vi "WHD_VEten_0.1.3.WS_BIDIR_Calibr_2.vi"() -> ()   [LabVIEW 2015]
uses:
  <vilib>/NI_Real-Time Target Support.lvlib
  <vilib>/rvi/interface/nirviReadWriteControl/nirviReadWriteControl.xnode
  <vilib>/rvi/interface/nirviMethod/nirviMethod.xnode
  <vilib>/rvi/interface/nirviOpenFPGA/nirviOpenFPGA.xnode
  <vilib>/rvi/interface/nirviCloseFPGA/nirviCloseFPGA.xnode
  <vilib>/userdefined/High Color/nirio_resource_hc.ctl
  <vilib>/rvi/errors/niLvFpgaMergeErrorWithErrorCode.vi
  <vilib>/Utility/file.llb/Write Delimited Spreadsheet (string).vi
  <vilib>/RTwatchdog.llb/Watchdog expiration actions.ctl
  AURA_Wheel/Json2Labv.lvlib
  AURA_Wheel/AuraWheelAPI/AuraWheel.lvlib
  <vilib>/rvi/errors/niLvFpgaAdjustHostInterfaceError.vi
  NiFpgaLv.dll
  <vilib>/Utility/error.llb/Error Cluster From Error Code.vi
  <vilib>/LabVIEW Targets/FPGA/cRIO/shared/nicrio_ModuleControls/nicrio_cRIO-9234_DataRatesRing2.ctl
  <vilib>/FPGAPlugInAG/cRIO-9031/niLvFpga_Run_cRIO-9031.vi
  <vilib>/FPGAPlugInAG/cRIO-9031/niLvFpga_Reset_cRIO-9031.vi
  FPGA Bitfiles/W&RDArabia_FPGATarget_FPGA8a2wsBIdirec_yJvL9yuTbZw.lvbitx
  <vilib>/Utility/config.llb/NI_LVConfig.lvlib
  <vilib>/Utility/config.llb/Write Key (Double).vi
  <vilib>/FPGAPlugInAG/cRIO-9031/niLvFpga_Open_cRIO-9031.vi
  <vilib>/FPGAPlugInAG/cRIO-9031/niLvFpga_ConfigureFifo_cRIO-9031.vi
  <vilib>/FPGAPlugInAG/cRIO-9031/niLvFpga_StartFifo_cRIO-9031.vi
  <vilib>/FPGAPlugInAG/cRIO-9031/niLvFpga_ReadFifo_cRIO-9031.vi
  <vilib>/FPGAPlugInAG/cRIO-9031/niLvFpga_StopFifo_cRIO-9031.vi
  <vilib>/FPGAPlugInAG/cRIO-9031/niLvFpga_Close_cRIO-9031.vi
panel:
  in  "Developer commad":string
  out "Save calibration":bool
  out "calibration log":path
  out "Pattern amplitude (g)":dbl=1.02
  out "Pattern frequency (Hz)":dbl=159.2
  out "Folder":path
  out "Report":string
  out "path calib":path
  out "AURA wheel test":bool
  out "LOG.txt":path
  out "Report_AURA":string
  out "RFID_Error":errorcluster
  out "error FPGA":errorcluster
  out "error AURA":errorcluster
  out "error manipulacion archivos":errorcluster
  out "Response headers":string
  out "Max RMS Ruedas":dbl[][](array[numeric])
  out "TAGs LR6":string[](array[string])
  out "TAGs HEX":string[](array[string])
  out "Parar":bool
  out "result":bool
  out "TAGs":string[](array[string])
  out "Temperatura (ºC)":dbl
  out "V (m/s)":dbl
  out "Digital?":bool=TRUE
  out "Watchdog config":T1={"reset system"=FALSE, "restart LabVIEW Runtime"=FALSE, "occurrence"=FALSE, "trigger protocol"=enum."active high", "trigger line"=enum."none", "disable watchdog on VI exit"=TRUE}
  out "Tiempo de adquisicion":dbl=10.0
  out "Adquirir":bool
  out "Nº Ruedas 1":i32
  out "NºRuedas 2":i32
  out "Disco Duro Disponible (bytes)":i64
  out "Buffer Overflow":bool
  out "Buffer Underflow":bool
  out "Archivo\nvalido?":bool
  out "Número de ejes detectados":i32
  out "Ejes_convoy":i32
  out "Tiempo de paso (s)":dbl
  out "created path":path
  out "Nombre de archivo":path[](array[path])
  out "LR6 IP address":string="192.168.106.94"
  out "Port LR6":u16=2001
  out "T fuera rango":bool
  out "Frecuencia de muestreo (Hz)":dbl=25600.0
  out "Escaneos de la FIFO por canal":u32=5000
  out "Tiempo extra al detector de paso (s)":dbl=1.0
  out "dt RMS":dbl=256.0
  out "Frecuencia de muestreo y módulo CRIO":T2=2 items=["51.200 kS/s (NI 9234)"=1, "25.600 kS/s (NI 9234)"=2, "17.067 kS/s (NI 9234)"=3, "12.800 kS/s (NI 9234)"=4, "10.240 kS/s (NI 9234)"=5, "8.533 kS/s (NI 9234)"=6, "7.314 kS/s (NI 9234)"=7, "6.400 kS/s (NI 9234)"=8, "5.689 kS/s (NI 9234)"=9, "5.120 kS/s (NI 9234)"=10, "4.654 kS/s (NI 9234)"=11, "4.267 kS/s (NI 9234)"=12, "3.938 kS/s (NI 9234)"=13, "3.657 kS/s (NI 9234)"=14, "3.413 kS/s (NI 9234)"=15, "3.200 kS/s (NI 9234)"=16, "3.012 kS/s (NI 9234)"=17, "2.845 kS/s (NI 9234)"=18, "2.695 kS/s (NI 9234)"=19, "2.560 kS/s (NI 9234)"=20, "2.438 kS/s (NI 9234)"=21, "2.328 kS/s (NI 9234)"=22, "2.226 kS/s (NI 9234)"=23, "2.133 kS/s (NI 9234)"=24, "2.048 kS/s (NI 9234)"=25, "1.969 kS/s (NI 9234)"=26, "1.896 kS/s (NI 9234)"=27, "1.829 kS/s (NI 9234)"=28, "1.765 kS/s (NI 9234)"=29, "1.707 kS/s (NI 9234)"=30, "1.652 kS/s (NI 9234)"=31]
  out "Puerto RFID":u16=2189
  out "IP RFID":string="192.168.106.99"
  out "Offset_rueda WS 2":fxp<+/-,24,-4>=0.004999998956918716 format="%.27g"
  out "Count(mSec)":u32=2
  out "RFID NEM on?":bool
  out "RFID LR6 on?":bool
  out "Canal cero WS1?":bool
  out "Canal cero WS2":bool
  out "Inicio pasada 2":timestamp
  in  "Calibration":bool
  out "Direccion 0?":bool
  out "Boton Adquirir?":bool
  out "RuedaDetectada2?":bool=TRUE
  out "RuedaDetectada1?":bool=TRUE
  out "Timeout ruedas":dbl
  out "Borrar archivos\nadquisicion con error":bool
  out "Able watchdog?":bool
  out "Reset watchdog?":bool
  out "Leer config RFID NEM":bool
  out "bytes to read":i32
  out "DeviceAddress":u8
  out "timeout ms (60000)":i32
  out "Max archivos":u32=2
  out "Bytes libre despues de borrar":u32=2
  out "Bytes min libre":u32=2
  out "Nº de acelerómetros":i32
  out "Nº inductivos":i32
  out "Offset_rueda WS 1":fxp<+/-,24,-4>=0.004999998956918716 format="%.27g"
  out "TAGs_AURAwheel":string[][](array[string])
  out "Plataformas?":bool
  out "Nº Ejes":i32[](array[numeric])
  out "Nº UTs":i32
  out "it-read-LR6":i32[](array[numeric])
  out "it-LR6":i32
  out "RFID_LR6_Error":errorcluster
  out "Series_flota":string[](array[string])
  out "Tabla_flota":string[][](array[string])
  out "Puntos medios de las ventanas":dbl[][](array[numeric])
  out "configuration file path":path=path "c:/Parametros.cfg"
  out "IP synchr":string
  out "data":cluster{"status":string}
  out "confRFID":path=path "c:/RFID/TAGS.csv"
  out "TAGS leidos":path=path "c:/RFID/TAGS.csv"
  out "Use Aura?":bool
  out "Parametros AuraWheel":string[](array[string])
  out "Parámetros acelerómetros":dbl[](array[numeric])
  out "Fin":bool
  out "Contador":i32=1
  out "Path LOG":path=path "c:/TEST"
  out "Fallo fotocelula":bool
  out "Path_Borrar":path=path "c:/Trenes"
  out "Longitud de la unidad":dbl
  out "Aviso no detección":string
  out "Time to Acquire Block (ms)":i32
  out "Distancia de acelerómetros":dbl[](array[numeric])
  out "Block Size":u32
  out "Distancias generales":dbl[](array[numeric])
  out "Reset del controlador":bool
  out "Parar la aplicación":bool
  out "date/time string":string
  out "Timeout ruedas":bool
  out "Tiempo":dbl
  out "Inicio pasada":timestamp
  out "Ultimo TEST":timestamp
  out "Fuente":bool=TRUE
  out "RFID_ID":refnum<k5>
  out "DC OK":string
  out "Aviso temperatura":string
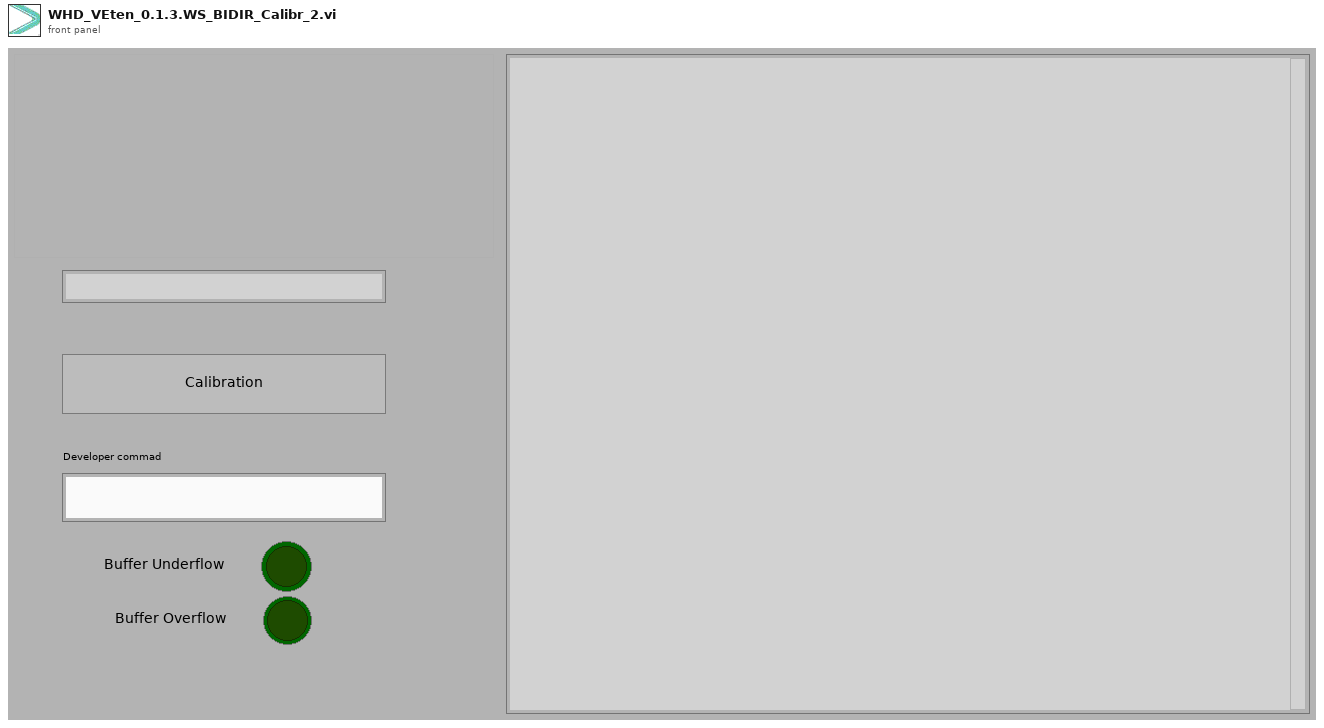
[diagram p1: front panel]
types:
  T1 = typedef "Watchdog expiration actions.ctl" = cluster{"reset system":bool, "restart LabVIEW Runtime":bool, "occurrence":bool, "trigger protocol":enum16{"active high", "active low", "open collector"}, "trigger line":enum16{"none", "line 0", "line 1", "line 2", "line 3", "line 4", "line 5", "line 6", "line 7", "SMB line 0"}, "disable watchdog on VI exit":bool}
  T2 = typedef "nicrio_cRIO-9234_DataRatesRing2.ctl" = u8
  T3 = typedef "nirio_resource_hc.ctl" = tag
  T4 = enum16{"Standard", "Buffered", "CRLF", "Immediate"}
  T5 = enum16{"open", "replace", "create", "open or create", "replace or create", "replace or create with confirmation"}
  T6 = enum16{"big-endian, network order", "native, host order", "little-endian"}
  T7 = cluster{"error IO":errorcluster, bool[], u32[], string[], dbl[]}
  T8 = cluster{"error out":errorcluster, dbl[], "TAGs":string[], "Direccion 0?":bool}
  T9 = cluster{"g_ts":dbl, "p_sp":dbl, "p_tp":dbl, "p_tg":cluster{"tg_n":dbl, "tg_t":string}[], "p_ax":cluster{"ax_n":dbl, "ax_sp":dbl, "ax_wh":cluster{"wh_p":dbl, "wh_a1":dbl, "wh_a2":dbl, "wh_a3":dbl, "wh_a4":dbl}[]}[]}
  T10 = cluster{"Frecuencia de muestreo y módulo CRIO":T2, "Count(mSec)":u32, "Frecuencia de muestreo (Hz)":dbl, "Escaneos de la FIFO por canal":u32, "Nº inductivos":i32, "Nº de acelerómetros":i32}
  T11 = typedef "NI_LVConfig.lvlib/Config Data RefNum.ctl" = refnum<k1>
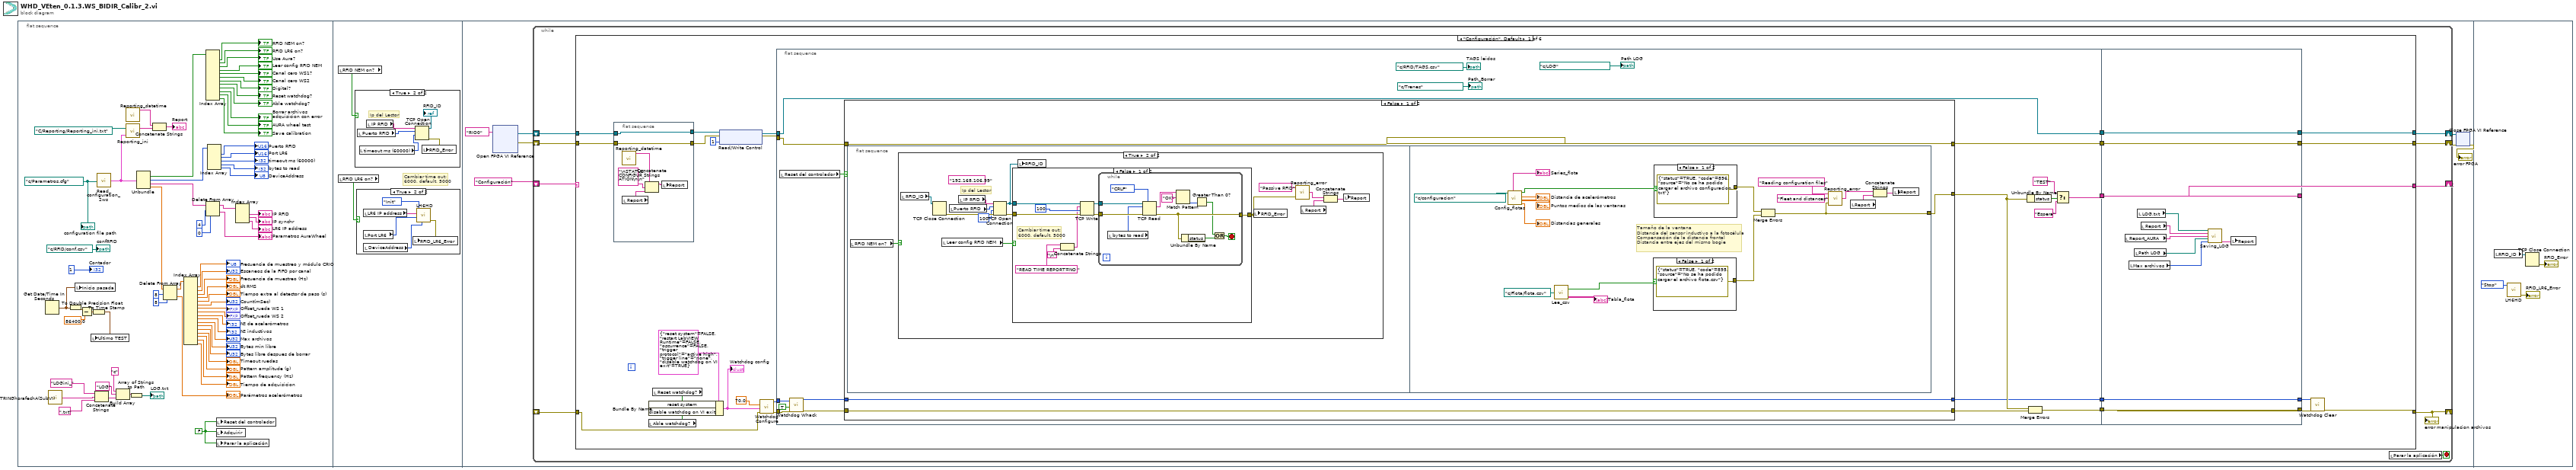
[diagram p0: block diagram]
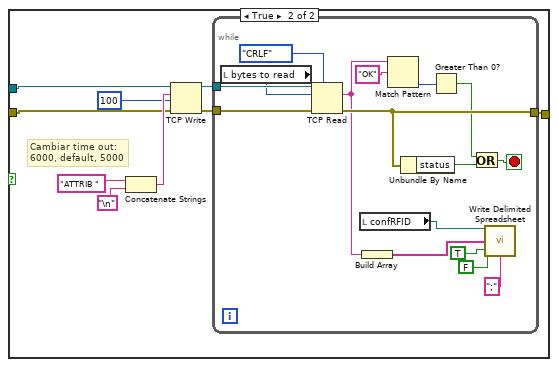
[diagram p5: hidden frame]
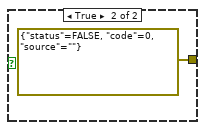
[diagram p6: hidden frame]
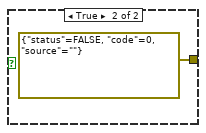
[diagram p7: hidden frame]
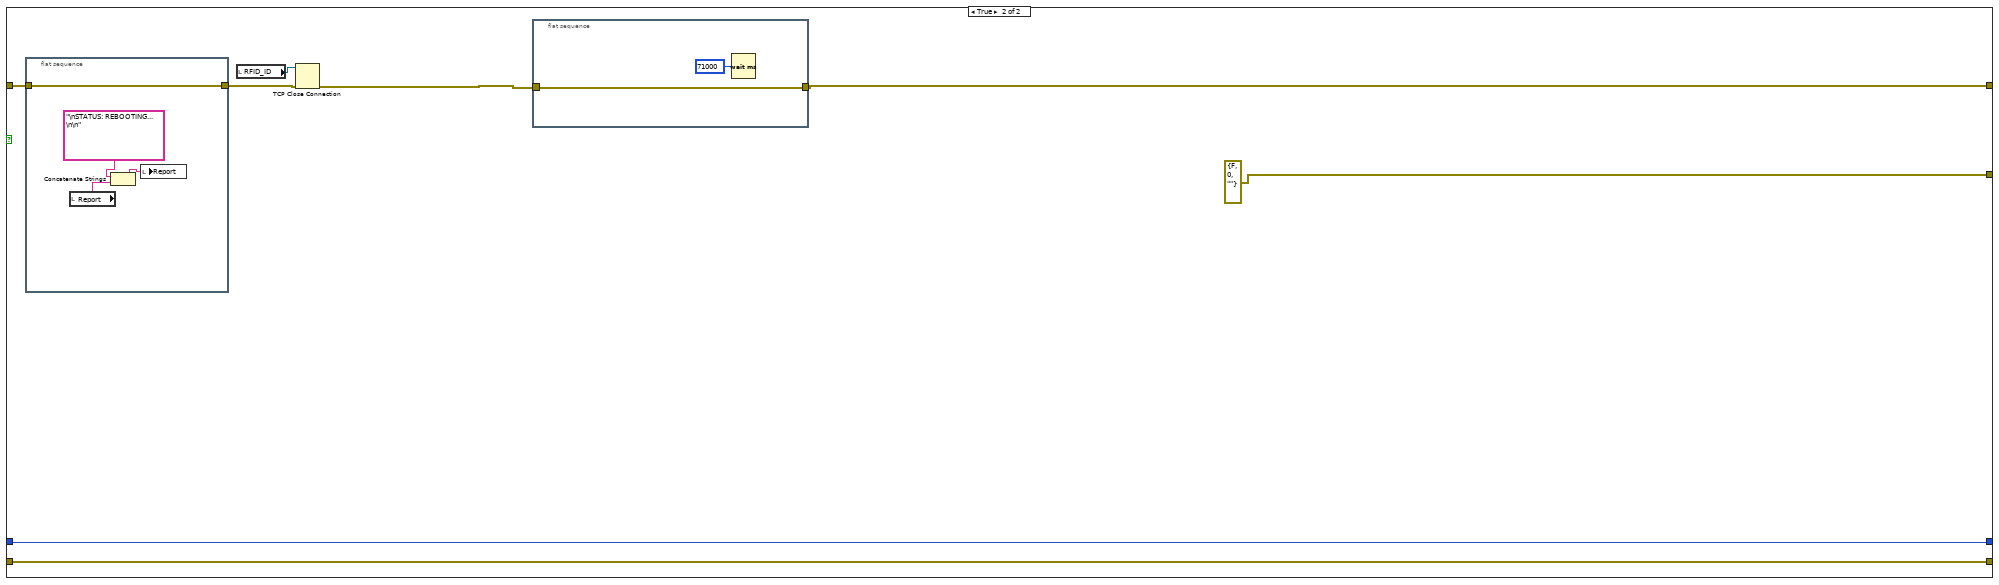
[diagram p8: hidden frame]
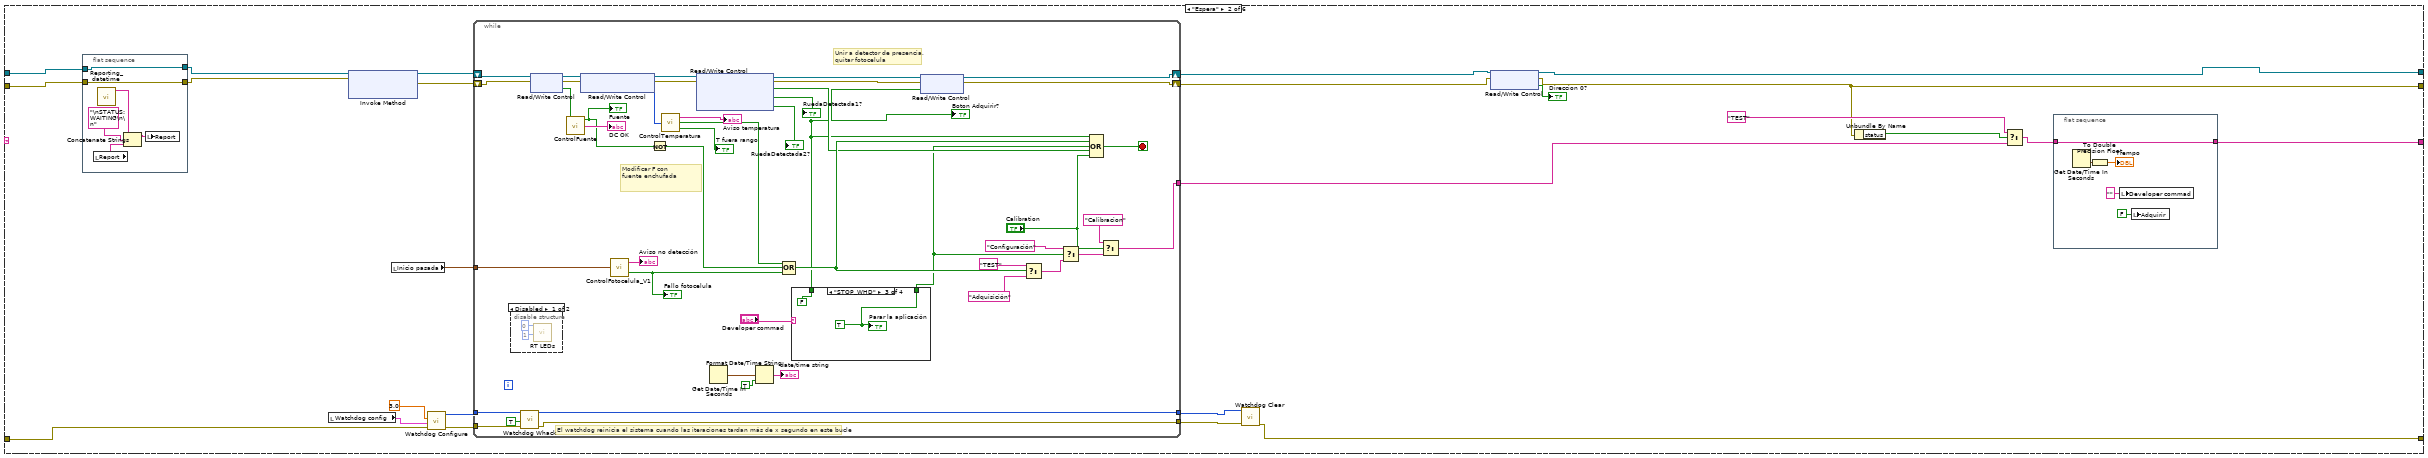
[diagram p9: hidden frame]
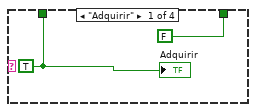
[diagram p10: hidden frame]
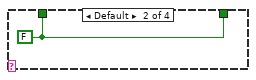
[diagram p11: hidden frame]
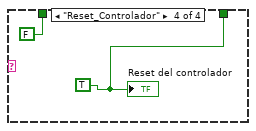
[diagram p12: hidden frame]
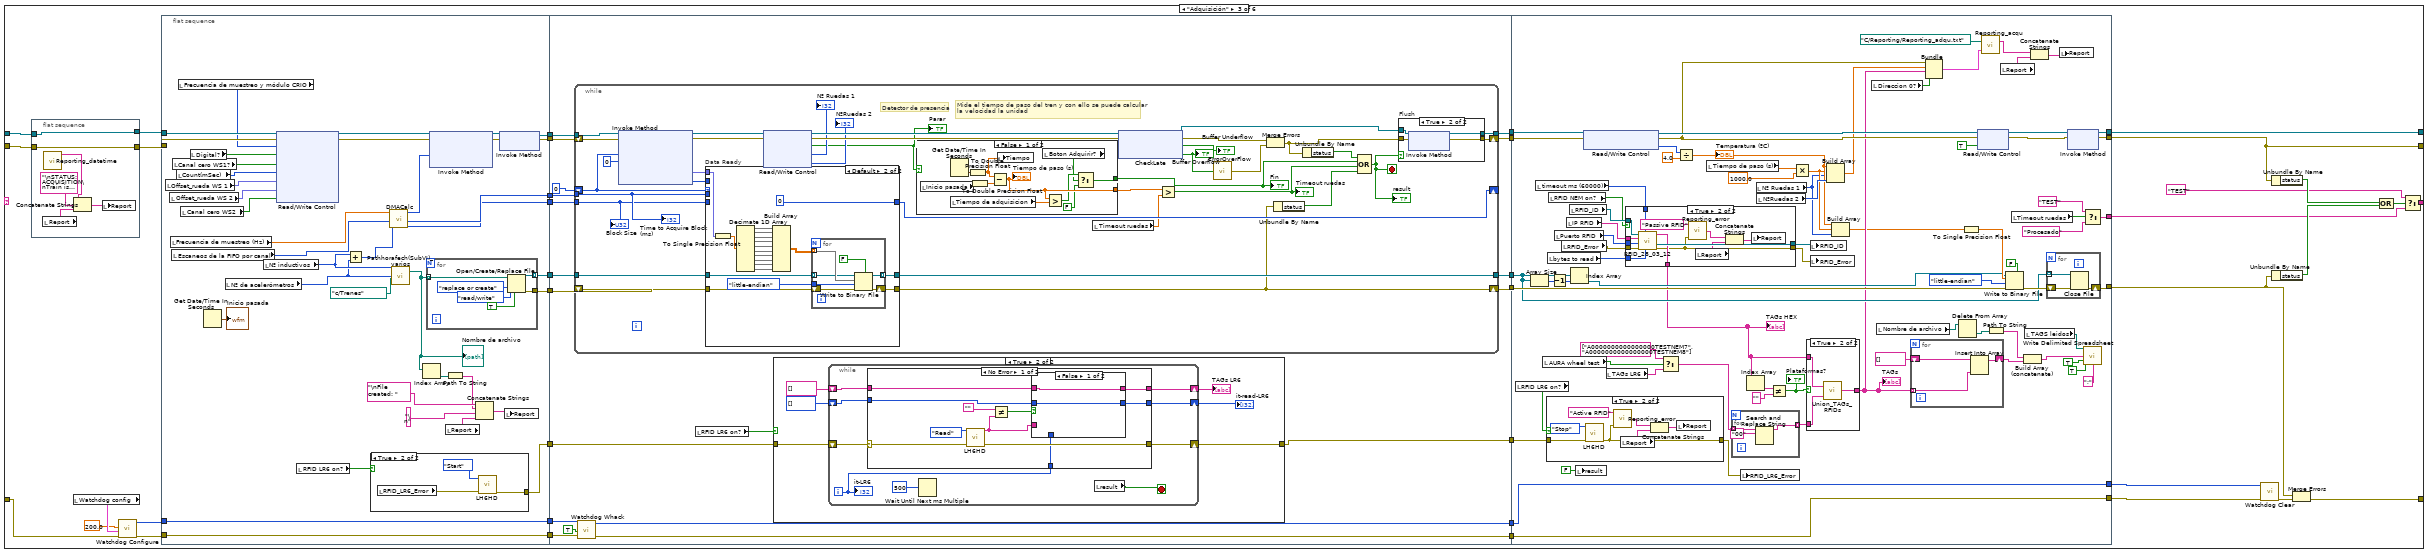
[diagram p14: hidden frame]
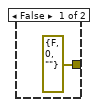
[diagram p15: hidden frame]
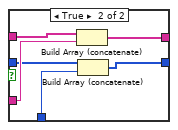
[diagram p17: hidden frame]
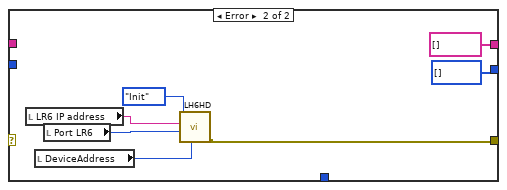
[diagram p18: hidden frame]
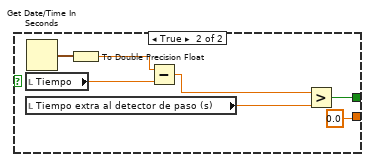
[diagram p19: hidden frame]
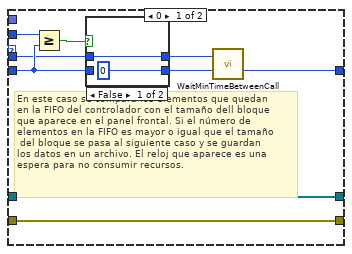
[diagram p20: hidden frame]
diagram:
  n1 = flat-sequence {
    frame #0 {
      w1 = FALSE ("Reset del controlador")
      w63 = path "c:/Parametros.cfg" ("configuration file path")
      n2 = Get Date/Time In Seconds() -> (seconds since 1Jan1904=w68:timestamp)
      n3 = call "STRINGhorafechA(SubVI).vi"() -> ("STRINGhora_fecha"=w12:string)
      n4 = To Double Precision Float(number=w68) -> (double precision float=w70:dbl)
      n5 = local write "Inicio pasada"(w68) -> ()
      n6 = Subtract(x=w70, y=86400.0) -> (x-y=w69:dbl)
      n7 = To Time Stamp(1:w69) -> (0:w67:timestamp)
      n8 = local write "Ultimo TEST"(w67) -> ()
      n9 = Concatenate Strings("LOGini_" ("string"), w12, ".txt" ("string")) -> (w14:string)
      n10 = call "Read_configuration_2ws.vi"("configuration file path"=w63) -> ("output cluster"=w18:T7)
      n11 = Build Array("c", "LOG" ("element"), w14) -> (w11:string[])
      n12 = call "Reporting_ini.vi"("Configuration cluster"=w18, "address repoting"=path "C:/Reporting/Reporting_ini.txt" ("file (use dialog)")) -> ("Reporting"=w17:string)  [unwired: 1 in]
      n13 = call "Reporting_datetime.vi"() -> ("String"=w15:string)  [unwired: 11 in]
      n14 = Array of Strings to Path(0:w11) -> (2:→"LOG.txt":path)  [unwired: 1 out]
      n15 = Unbundle(w18) -> (w66:bool[], w65:u32[], w58:string[], w62:dbl[])  [unwired: 1 out]
      n16 = Concatenate Strings(w15, w17) -> (→"Report":string)
      n17 = Delete From Array(array=w62, length=8, index=8) -> (deleted portion=→"Parámetros acelerómetros":dbl[], array with subset deleted=w61:dbl[])
      n18 = Index Array(array=w61) -> (element #1=→"Frecuencia de muestreo y módulo CRIO":dbl, element #2=→"Escaneos de la FIFO por canal":dbl, element #3=→"Frecuencia de muestreo (Hz)":dbl, element #4=→"dt RMS":dbl, element #5=→"Tiempo extra al detector de paso (s)":dbl, element #6=→"Count(mSec)":dbl, element #7=→"Offset_rueda WS 1":dbl, element #8=→"Offset_rueda WS 2":dbl, element #9=→"Nº de acelerómetros":dbl, element #10=→"Nº inductivos":dbl, element #11=→"Max archivos":dbl, element #12=→"Bytes min libre":dbl, element #13=→"Bytes libre despues de borrar":dbl, element #14=→"Timeout ruedas":dbl, element #15=→"Pattern amplitude (g)":dbl, element #16=→"Pattern frequency (Hz)":dbl, element #17=→"Tiempo de adquisicion":dbl)  [unwired: 17 in]
      n19 = Index Array(array=w66) -> (element #1=→"RFID NEM on?":bool, element #2=→"RFID LR6 on?":bool, element #3=→"Use Aura?":bool, element #4=→"Leer config RFID NEM":bool, element #5=→"Canal cero WS1?":bool, element #6=→"Canal cero WS2":bool, element #7=→"Digital?":bool, element #8=→"Reset watchdog?":bool, element #9=→"Able watchdog?":bool, element #10=→"Borrar archivos\nadquisicion con error":bool, element #11=→"AURA wheel test":bool, element #12=→"Save calibration":bool)  [unwired: 12 in]
      n20 = Delete From Array(array=w58, length=4, index=0) -> (deleted portion=→"Parametros AuraWheel":string[], array with subset deleted=w57:string[])
      n21 = Index Array(array=w65) -> (element #1=→"Puerto RFID":u32, element #2=→"Port LR6":u32, element #3=→"timeout ms (60000)":u32, element #4=→"bytes to read":u32, element #5=→"DeviceAddress":u32)  [unwired: 5 in]
      n22 = local write "Reset del controlador"(w1) -> ()
      n23 = local write "Adquirir"(w1) -> ()
      n24 = local write "Parar la aplicación"(w1) -> ()
      n25 = Index Array(array=w57) -> (element #1=→"IP RFID":string, element #2=→"IP synchr":string, element #3=→"LR6 IP address":string)  [unwired: 3 in]
      "Contador" <- 1
      "confRFID" <- path "c:/RFID/conf.csv" ("file path (use dialog)")
      "configuration file path" <- w63
    }
    frame #1 {
      # "Cambiar time out:\n6000, default, 5000"
      n26 = local read "RFID NEM on?"() -> (w73:bool)
      n27 = local read "RFID LR6 on?"() -> (w72:bool)
      n28 = case shown="True" w73 {
        frame False {
        }
        frame True {
          # "Ip del Lector"
          n29 = local read "Puerto RFID"() -> (w81:u16)
          n30 = local read "timeout ms (60000)"() -> (w79:i32)
          n31 = local read "IP RFID"() -> (w82:string)
          n32 = TCP Open Connection(address=w82, remote port or service name=w81, timeout ms (60000)=w79) -> (connection ID=→"RFID_ID":refnum<k5>, error out=w80:errorcluster)  [unwired: 1 in, 1 out]
          n33 = local write "RFID_Error"(w80) -> ()
        }
      }
      n34 = case shown="True" w72 {
        frame False {
        }
        frame True {
          n35 = local read "LR6 IP address"() -> (w74:string)
          n36 = local read "Port LR6"() -> (w75:u16)
          n37 = local read "DeviceAddress"() -> (w76:u8)
          n38 = call "LH6HD.vi"("DeviceAddress"=w76, "Reader Port"=w75, "IP Address"=w74, "Action"=enum16{"Init", "Start", "Read", "Stop", "Exit"}."Init") -> ("error out"=w78:errorcluster)  [unwired: 6 in, 1 out]
          n39 = local write "RFID_LR6_Error"(w78) -> ()
        }
      }
    }
    frame #2 {
      n40 = xnode "Open FPGA VI Reference"("resource name"=T3 "RIO0") -> ("FPGA VI Reference Out"=w90:refnum<k20>, "error out"=w89:errorcluster)  [unwired: 1 in]
      n41 = while {
        shift-right: [w91] -> _
        shift-left: "Configuración" -> [w99]
        shift-right: [w93] -> w86
        shift-left: w90 -> [w98]
        shift-right: [w92] -> w85
        shift-left: w89 -> [w97]
        shift-right: [w96] -> _
        shift-left: _ -> [w95]
        stop <- w94 stop-if-true
        n42 = case shown="\"Configuración\", Default" w99 {
          tunnel: [w114 w278 w368 w725 w973 "Espera"] -> w91
          tunnel: [w124 w266 w382 w714 w972 w1046] -> w93
          tunnel: [w125 w265 w383 w712 w971 w1045] -> w92
          tunnel: w98 -> [w108 w264 w354 w715 w972 w1051]
          tunnel: w97 -> [w107 w263 w353 w713 w964 w1050]
          tunnel: [w121 w272 w380 w710 w963 _] -> w96
          tunnel: w95 -> [w113 w277 w364 w724 w960 _]
          frame "Configuración", Default {
            n43 = flat-sequence {
              tunnel: w108 -> [w131]
              tunnel: w107 -> [w130]
              tunnel: [w131] -> w106
              tunnel: [w130] -> w105
              frame #0 {
                n44 = call "Reporting_datetime.vi"() -> ("String"=w126:string)  [unwired: 11 in]
                n45 = local read "Report"() -> (w127:string)
                n46 = Concatenate Strings(w126, "\nSTATUS: CONFIGURATION\n\n", w127) -> (w129:string)
                n47 = local write "Report"(w129) -> ()
              }
            }
            n48 = local read "Able watchdog?"() -> (w118:bool)
            n49 = local read "Reset watchdog?"() -> (w119:bool)
            n50 = Bundle By Name(cluster=T1 {"reset system"=FALSE, "restart LabVIEW Runtime"=FALSE, "occurrence"=FALSE, "trigger protocol"=enum."active high", "trigger line"=enum."none", "disable watchdog on VI exit"=TRUE} ("expiration actions"), "reset system"=w119, "disable watchdog on VI exit"=w118) -> (w112:T1)
            "Watchdog config" <- w112
            n51 = xnode "Read/Write Control"("FPGA VI Reference In"=w106, "error in"=w105, "Cycles to Filter"=u16 1) -> ("FPGA VI Reference Out"=w117:refnum<k20>, "error out"=w116:errorcluster)
            n52 = call <vilib>:"Watchdog Configure.vi"("error in (no error)"=w113, "expiration actions"=w112, "timeout (1 sec)"=70.0) -> ("error out"=w109:errorcluster, "watchdogID"=w110:u64)  [unwired: 1 in, 2 out]
            n53 = flat-sequence {
              tunnel: w117 -> [w143]
              tunnel: w116 -> [w140]
              tunnel: w110 -> [w133]
              tunnel: w109 -> [w132]
              tunnel: [w142] -> w104
              tunnel: [w150] -> w103
              tunnel: [w143] -> w102
              tunnel: [w145] -> w101
              tunnel: [w137] -> w100
              tunnel: [w256] -> w123
              tunnel: [w257] -> w122
              tunnel: [w258] -> w124
              tunnel: [w259] -> w114
              tunnel: [w260] -> w125
              tunnel: w104 -> [w260]
              tunnel: w103 -> [w259]
              tunnel: w102 -> [w258]
              tunnel: w101 -> [w257]
              tunnel: w100 -> [w256]
              frame #0 {
                n54 = local read "Reset del controlador"() -> (w139:bool)
                n55 = call <vilib>:"Watchdog Whack.vi"("error in (no error)"=w132, "reset watchdog after expire? (F)"=TRUE, "watchdogID in"=w133) -> ("error out"=w135:errorcluster, "watchdogID out"=w136:u64)  [unwired: 2 in, 1 out]
                n56 = case shown="False" w139 {
                  tunnel: w140 -> [w155 w238]
                  tunnel: [w155 w241] -> w142
                  tunnel: [w152 errorcluster {"status"=FALSE, "code"=0, "source"=""} ("error IO")] -> w141
                  tunnel: [w154 w240] -> w137
                  tunnel: w136 -> [w154 w240]
                  tunnel: w135 -> [w153 w239]
                  tunnel: [w153 w239] -> w134
                  frame False {
                    n57 = flat-sequence {
                      tunnel: [w215] -> w152
                      frame #0 {
                        n58 = local read "RFID NEM on?"() -> (w156:bool)
                        n59 = case shown="True" w156 {
                          frame False {
                          }
                          frame True {
                            (unwired) "192.168.106.99" ("address")
                            # "Ip del Lector"
                            n60 = local read "RFID_ID"() -> (w168:refnum<k5>)
                            n61 = TCP Close Connection(connection ID=w168) -> (error out=w169:errorcluster)  [unwired: 2 in, 1 out]
                            n62 = local read "Leer config RFID NEM"() -> (w162:bool)
                            n63 = local read "Puerto RFID"() -> (w166:u16)
                            n64 = local read "IP RFID"() -> (w165:string)
                            n65 = TCP Open Connection(address=w165, remote port or service name=w166, timeout ms (60000)=100, error in (no error)=w169) -> (connection ID=w167:refnum<k5>, error out=w163:errorcluster)  [unwired: 1 out]
                            n66 = case shown="False" w162 {
                              tunnel: w167 -> [w178 w192]
                              tunnel: [w176 w190] -> w161
                              tunnel: w163 -> [w173 w191]
                              frame False {
                                # "Cambiar time out:\n6000, default, 5000"
                                n67 = Concatenate Strings("READ TIME REPORT=NO " ("data in"), "\n") -> (w170:string)
                                n68 = TCP Write(connection ID=w178, data in=w170, error in (no error)=w173, 9:100 ("timeout ms (25000)")) -> (connection ID out=w174:refnum<k5>, error out=w175:errorcluster)  [unwired: 1 out]
                                n69 = while {
                                tunnel: w175 -> [w188]
                                tunnel: w174 -> [w187]
                                tunnel: [w186] -> w176
                                stop <- w183 stop-if-true
                                n70 = local read "bytes to read"() -> (w179:i32)
                                n71 = TCP Read(connection ID=w187, bytes to read=w179, error in (no error)=w188, 7:T4."CRLF" ("mode (standard)")) -> (data out=w181:string, error out=w186:errorcluster)  [unwired: 1 in, 1 out]
                                n72 = Match Pattern(string=w181, regular expression="OK") -> (offset past match=w184:i32)  [unwired: 4 out]
                                n73 = Unbundle By Name(w186) -> ("status"=w182:bool)
                                n74 = Greater Than 0?(x=w184) -> (x > 0?=w180:bool)
                                n75 = Or(x=w180, y=w182) -> (x .or. y?=w183:bool)
                                }
                              }
                              frame True {
                                # "Cambiar time out:\n6000, default, 5000"
                                n76 = Concatenate Strings("ATTRIB " ("data in"), "\n") -> (w198:string)
                                n77 = TCP Write(connection ID=w192, data in=w198, error in (no error)=w191, 9:100 ("timeout ms (25000)")) -> (connection ID out=w195:refnum<k5>, error out=w194:errorcluster)  [unwired: 1 out]
                                n78 = while {
                                tunnel: w194 -> [w213]
                                tunnel: w195 -> [w212]
                                tunnel: [w211] -> w190
                                stop <- w208 stop-if-true
                                n79 = local read "bytes to read"() -> (w199:i32)
                                n80 = TCP Read(connection ID=w212, bytes to read=w199, error in (no error)=w213, 7:T4."CRLF" ("mode (standard)")) -> (data out=w202:string, error out=w211:errorcluster)  [unwired: 1 in, 1 out]
                                n81 = local read "confRFID"() -> (w201:path)
                                n82 = Build Array(w202) -> (w200:string[])
                                n83 = Match Pattern(string=w202, regular expression="OK") -> (offset past match=w209:i32)  [unwired: 4 out]
                                n84 = Unbundle By Name(w211) -> ("status"=w207:bool)
                                n85 = Greater Than 0?(x=w209) -> (x > 0?=w206:bool)
                                n86 = Or(x=w206, y=w207) -> (x .or. y?=w208:bool)
                                n87 = call-poly <vilib>:"Write Delimited Spreadsheet.vi"("file path (dialog if empty)"=w201, "1D data"=w200, "append to file? (new file:F)"=FALSE ("transpose? (no:F)"), "transpose? (no:F)"=TRUE ("append to file? (new file:F)"), "delimiter (\\t)"=";" ("delimiter (\\t)")) -> ()  [unwired: 9 in, 2 out]
                                }
                              }
                            }
                            n88 = local write "RFID_ID"(w167) -> ()
                            n89 = local write "RFID_Error"(w161) -> ()
                            n90 = call "Reporting_error.vi"("error out 2"=w161, "Concept"="Passive RFID") -> ("Reporting"=w158:string)  [unwired: 1 in]
                            n91 = local read "Report"() -> (w159:string)
                            n92 = Concatenate Strings(w158, w159) -> (w157:string)
                            n93 = local write "Report"(w157) -> ()
                          }
                        }
                      }
                      frame #1 {
                        # "Tamaño de la ventana\nDistancia del sensor inductivo a la fotocélula\nCompensación de la distancia frontal\nDistancia entre ejes del mismo bogie"
                        n94 = call "Config_flotas.vi"("file path (dialog if empty)"=path "c:/configuracion") -> ("Distancias generales"=→"Distancias generales":dbl[], "Puntos medios de las ventanas"=→"Puntos medios de las ventanas":dbl[][], "Distancia de acelerómetros"=→"Distancia de acelerómetros":dbl[], "Distacias y medidas de dispositivos"=w228:bool, "Series_flota"=→"Series_flota":string[])  [unwired: 3 in]
                        n95 = call "Lee_csv.vi"("Path"=path "c:/Flota/flota.csv") -> ("Tabla_flota"=→"Tabla_flota":string[][], "Lectura_OK?"=w225:bool)
                        n96 = case shown="False" w225 {
                          tunnel: [errorcluster {"status"=TRUE, "code"=895, "source"="No se ha podido cargar el archivo flota.csv"} ("error out") errorcluster {"status"=FALSE, "code"=0, "source"=""} ("error out")] -> w229
                          frame False {
                          }
                          frame True {
                          }
                        }
                        n97 = case shown="False" w228 {
                          tunnel: [errorcluster {"status"=TRUE, "code"=896, "source"="No se ha podido cargar el archivo configuracion.txt"} ("error out") errorcluster {"status"=FALSE, "code"=0, "source"=""} ("error out")] -> w230
                          frame False {
                          }
                          frame True {
                          }
                        }
                        n98 = Merge Errors(w230, w229) -> (w215:errorcluster)
                        n99 = call "Reporting_error.vi"("error out 2"=w215, "Concept explanation"="Fleet and distances", "Concept"="Reading configuration files") -> ("Reporting"=w217:string)
                        n100 = local read "Report"() -> (w216:string)
                        n101 = Concatenate Strings(w217, w216) -> (w218:string)
                        n102 = local write "Report"(w218) -> ()
                      }
                    }
                  }
                  frame True {
                    n103 = flat-sequence {
                      tunnel: w238 -> [w247]
                      tunnel: [w247] -> w237
                      frame #0 {
                        n104 = local read "Report"() -> (w246:string)
                        n105 = Concatenate Strings("\nSTATUS: REBOOTING...\n\n", w246) -> (w244:string)
                        n106 = local write "Report"(w244) -> ()
                      }
                    }
                    n107 = local read "RFID_ID"() -> (w243:refnum<k5>)
                    n108 = TCP Close Connection(connection ID=w243, error in (no error)=w237) -> (error out=w236:errorcluster)  [unwired: 2 out]
                    n109 = flat-sequence {
                      tunnel: [w249] -> w241
                      tunnel: w236 -> [w249]
                      frame #0 {
                        n110 = Wait (ms)(milliseconds to wait=u32 71000) -> ()  [unwired: 1 out]
                      }
                    }
                  }
                }
                n111 = Unbundle By Name(w141) -> ("status"=w151:bool)
                n112 = Merge Errors(w141, w134) -> (w145:errorcluster)
                n113 = Select(t="TEST", s=w151, f="Espera") -> (s? t:f=w150:string)
                "Path_Borrar" <- path "c:/Trenes" ("file path (use dialog)")
                "Path LOG" <- path "c:/LOG" ("file path (use dialog)")
                "TAGS leidos" <- path "c:/RFID/TAGS.csv" ("file path (use dialog)")
              }
              frame #1 {
                n114 = local read "Report_AURA"() -> (w253:string)
                n115 = local read "Max archivos"() -> (w254:u32)
                n116 = local read "Path LOG"() -> (w255:path)
                n117 = local read "LOG.txt"() -> (w250:path)
                n118 = local read "Report"() -> (w252:string)
                n119 = call "Saving_LOG.vi"("Path"=w250, "Report"=w252, "Report AURA"=w253, "Path Carpeta"=w255, "Nº Archivos Max"=w254) -> ("Report"=w251:string)  [unwired: 9 in, 1 out]
                n120 = local write "Report"(w251) -> ()
              }
            }
            n121 = call <vilib>:"Watchdog Clear.vi"("error in (no error)"=w122, "watchdogID in"=w123) -> ("error out"=w121:errorcluster)  [unwired: 5 in]
          }
          frame "Espera" {
            n122 = flat-sequence {
              tunnel: w264 -> [w291]
              tunnel: w263 -> [w290]
              tunnel: [w291] -> w262
              tunnel: [w290] -> w261
              frame #0 {
                n123 = local read "Report"() -> (w287:string)
                n124 = call "Reporting_datetime.vi"() -> ("String"=w286:string)  [unwired: 11 in]
                n125 = Concatenate Strings(w286, "\nSTATUS: WAITING\n\n", w287) -> (w289:string)
                n126 = local write "Report"(w289) -> ()
              }
            }
            n127 = local read "Watchdog config"() -> (w271:T1)
            n128 = xnode "Invoke Method"("FPGA VI Reference In"=w262, "error in"=w261) -> ("FPGA VI Reference Out"=w281:refnum<k20>, "error out"=w280:errorcluster)  [unwired: 1 in]
            n129 = local read "Inicio pasada"() -> (w285:timestamp)
            n130 = call <vilib>:"Watchdog Configure.vi"("error in (no error)"=w277, "expiration actions"=w271, "timeout (1 sec)"=3.0) -> ("error out"=w276:errorcluster, "watchdogID"=w275:u64)  [unwired: 1 in, 2 out]
            n131 = while {
              tunnel: [w304] -> w284
              shift-right: [w313] -> w267
              shift-left: w281 -> [w321]
              shift-right: [w312] -> w268
              shift-left: w280 -> [w320]
              tunnel: w285 -> [w324]
              tunnel: w276 -> [w310]
              tunnel: w275 -> [w311]
              tunnel: [w309] -> w274
              tunnel: [w308] -> w273
              stop <- w302 stop-if-true
              # "Modificar F con\nfuente enchufada"
              # "Unir a detector de presencia,\nquitar fotocelula"
              # "El watchdog reinicia el sistema cuando las iteraciones tardan más de x segundo en este bucle"
              n132 = disable-structure shown="Disabled" {
                frame Disabled {
                  n133 = call <vilib>:"RT LEDs.vi"("State"=1, "LED Num"=0) -> ()  [unwired: 1 in, 5 out]
                }
                frame Enabled {
                }
              }
              n134 = call <vilib>:"Watchdog Whack.vi"("error in (no error)"=w310, "reset watchdog after expire? (F)"=TRUE, "watchdogID in"=w311) -> ("error out"=w308:errorcluster, "watchdogID out"=w309:u64)  [unwired: 2 in, 1 out]
              n135 = xnode "Read/Write Control"("FPGA VI Reference In"=w321, "error in"=w320) -> ("FPGA VI Reference Out"=w333:refnum<k20>, "error out"=w332:errorcluster, "DC OK"=w337:bool)
              n136 = call "ControlFuente.vi"("DC OK 3"=w337) -> ("DC OK 2"=w297:bool, "DC OK"=→"DC OK":string)  [unwired: 1 out]
              "Fuente" <- w297
              n137 = xnode "Read/Write Control"("FPGA VI Reference In"=w333, "error in"=w332) -> ("FPGA VI Reference Out"=w328:refnum<k20>, "error out"=w327:errorcluster, "Chassis Temperature"=w335:i16)
              n138 = call "ControlFotocelula_V1.vi"("Tiempo de entrada a espera"=w324) -> ("Aviso no detección"=→"Aviso no detección":string, "Boolean"=w325:bool)
              "Fallo fotocelula" <- w325
              n139 = Not(x=w297) -> (.not. x?=w298:bool)
              n140 = call "ControlTemperatura.vi"("Chassis Temperature"=w335) -> ("Aviso temperatura"=→"Aviso temperatura":string, "Boolean"=w329:bool, "T fuera rango"=→"T fuera rango":bool)
              n141 = xnode "Read/Write Control"("FPGA VI Reference In"=w328, "error in"=w327) -> ("FPGA VI Reference Out"=w323:refnum<k20>, "error out"=w322:errorcluster, "Detector de presencia"=w316:bool, "RuedaDetectada1?"=→"RuedaDetectada1?":bool, "RuedaDetectada2?"=→"RuedaDetectada2?":bool)
              n142 = Get Date/Time In Seconds() -> (seconds since 1Jan1904=w318:timestamp)
              n143 = Format Date/Time String(seconds (now)=w318, UTC format=TRUE) -> (date/time string=→"date/time string":string)  [unwired: 1 in]
              n144 = Compound Arithmetic op=OR(w329, w298, w325) -> (w326:bool)
              n145 = case shown="\"STOP_WHD\"" "Developer commad" {
                tunnel: [w343 w344 FALSE ("Adquirir") FALSE ("Adquirir")] -> w301
                tunnel: [FALSE ("Adquirir") w344 w345 w347] -> w300
                frame "Adquirir" {
                  w343 = TRUE ("Adquirir")
                  "Adquirir" <- w343
                }
                frame Default {
                  w344 = FALSE ("Adquirir")
                }
                frame "STOP_WHD" {
                  w345 = TRUE ("Adquirir")
                  "Parar la aplicación" <- w345
                }
                frame "Reset_Controlador" {
                  w347 = TRUE ("Adquirir")
                  "Reset del controlador" <- w347
                }
              }
              "Boton Adquirir?" <- w301
              n146 = xnode "Read/Write Control"("FPGA VI Reference In"=w323, "error in"=w322, "Fotocélula"=w301) -> ("FPGA VI Reference Out"=w313:refnum<k20>, "error out"=w312:errorcluster)
              n147 = Select(t="TEST", s=w326, f="Adquisición") -> (s? t:f=w338:string)
              n148 = Select(t="Configuración", s=w300, f=w338) -> (s? t:f=w306:string)
              n149 = Compound Arithmetic op=OR(w301, w326, w300, w316, "Calibration") -> (w302:bool)
              n150 = Select(t="Calibracion", s="Calibration", f=w306) -> (s? t:f=w304:string)
            }
            n151 = call <vilib>:"Watchdog Clear.vi"("error in (no error)"=w273, "watchdogID in"=w274) -> ("error out"=w272:errorcluster)  [unwired: 5 in]
            n152 = xnode "Read/Write Control"("FPGA VI Reference In"=w267, "error in"=w268) -> ("FPGA VI Reference Out"=w266:refnum<k20>, "error out"=w265:errorcluster, "Direccion 0?"=→"Direccion 0?":bool)
            n153 = Unbundle By Name(w265) -> ("status"=w283:bool)
            n154 = Select(t="TEST", s=w283, f=w284) -> (s? t:f=w279:string)
            n155 = flat-sequence {
              tunnel: [w295] -> w278
              tunnel: w279 -> [w295]
              frame #0 {
                n156 = Get Date/Time In Seconds() -> (seconds since 1Jan1904=w296:timestamp)
                n157 = To Double Precision Float(number=w296) -> (double precision float=→"Tiempo":dbl)
                n158 = local write "Developer commad"("" ("Developer commad")) -> ()
                n159 = local write "Adquirir"(FALSE ("Adquirir")) -> ()
              }
            }
          }
          frame "Adquisición" {
            n160 = flat-sequence {
              tunnel: w354 -> [w394]
              tunnel: w353 -> [w393]
              tunnel: [w394] -> w352
              tunnel: [w393] -> w351
              frame #0 {
                n161 = local read "Report"() -> (w390:string)
                n162 = call "Reporting_datetime.vi"() -> ("String"=w389:string)  [unwired: 11 in]
                n163 = Concatenate Strings(w389, "\nSTATUS: ACQUISITION\nTrain is passing\n\n", w390) -> (w392:string)
                n164 = local write "Report"(w392) -> ()
              }
            }
            n165 = local read "Watchdog config"() -> (w365:T1)
            n166 = call <vilib>:"Watchdog Configure.vi"("error in (no error)"=w364, "expiration actions"=w365, "timeout (1 sec)"=200.0) -> ("error out"=w362:errorcluster, "watchdogID"=w363:u64)  [unwired: 1 in, 2 out]
            n167 = flat-sequence {
              tunnel: w351 -> [w428]
              tunnel: w352 -> [w429]
              tunnel: [w427] -> w379
              tunnel: [w426] -> w378
              tunnel: [w425] -> w377
              tunnel: [w424] -> w376
              tunnel: [w423] -> w375
              tunnel: [w422] -> w374
              tunnel: [w412] -> w367
              tunnel: w363 -> [w411]
              tunnel: w362 -> [w410]
              tunnel: [w411] -> w361
              tunnel: [w410] -> w360
              tunnel: [w444] -> w388
              tunnel: [w461] -> w387
              tunnel: [w460] -> w386
              tunnel: [w459] -> w385
              tunnel: [w452] -> w384
              tunnel: w379 -> [w458]
              tunnel: w378 -> [w457]
              tunnel: w377 -> [w456]
              tunnel: w376 -> [w455]
              tunnel: w375 -> [w454]
              tunnel: w374 -> [w453]
              tunnel: w367 -> [w450]
              tunnel: [w449] -> w366
              tunnel: w361 -> [w448]
              tunnel: w360 -> [w447]
              tunnel: [w445] -> w359
              tunnel: w388 -> [w625]
              tunnel: w387 -> [w620]
              tunnel: w386 -> [w619]
              tunnel: w385 -> [w639]
              tunnel: [w666] -> w371
              tunnel: w384 -> [w668]
              tunnel: [w655] -> w381
              tunnel: [w656] -> w383
              tunnel: [w657] -> w382
              tunnel: w366 -> [w634]
              tunnel: w359 -> [w626]
              tunnel: [w626] -> w357
              tunnel: [w625] -> w356
              frame #0 {
                n168 = local read "Offset_rueda WS 1"() -> (w405:fxp<+/-,24,-4>)
                n169 = local read "Offset_rueda WS 2"() -> (w406:fxp<+/-,24,-4>)
                n170 = local read "Frecuencia de muestreo (Hz)"() -> (w420:dbl)
                n171 = local read "Escaneos de la FIFO por canal"() -> (w409:u32)
                n172 = local read "Canal cero WS1?"() -> (w414:bool)
                n173 = local read "Count(mSec)"() -> (w413:u32)
                n174 = local read "Frecuencia de muestreo y módulo CRIO"() -> (w416:T2)
                n175 = local read "Canal cero WS2"() -> (w404:bool)
                n176 = local read "Digital?"() -> (w415:bool)
                n177 = Get Date/Time In Seconds() -> (seconds since 1Jan1904=→"Inicio pasada":timestamp)
                n178 = local read "Nº de acelerómetros"() -> (w402:i32)
                n179 = local read "Nº inductivos"() -> (w403:i32)
                n180 = xnode "Read/Write Control"("FPGA VI Reference In"=w429, "error in"=w428, "Data Rate"=w416, "Digital?"=w415, "Canal cero WS1?"=w414, "Count(mSec)"=w413, "Offset_WS1"=w405, "Offset_WS2"=w406, "Canal cero WS2?"=w404) -> ("FPGA VI Reference Out"=w419:refnum<k20>, "error out"=w418:errorcluster)
                n181 = local read "RFID LR6 on?"() -> (w407:bool)
                n182 = Add(x=w403, y=w402) -> (x+y=w408:i32)
                n183 = case shown="True" w407 {
                  tunnel: [errorcluster {"status"=FALSE, "code"=0, "source"=""} ("error out") w434] -> w412
                  frame False {
                  }
                  frame True {
                    n184 = local read "RFID_LR6_Error"() -> (w435:errorcluster)
                    n185 = call "LH6HD.vi"("error in (no error)"=w435, "Action"=enum16{"Init", "Start", "Read", "Stop", "Exit"}."Start") -> ("error out"=w434:errorcluster)  [unwired: 8 in, 1 out]
                  }
                }
                n186 = call "DMACalc.vi"("Number of Channels"=w408, "Number of Samples"=w409, "Rate (Hz)"=w420) -> ("Block Size"=w424:u32, "Time to Acquire Block (ms)"=w425:i32, "Host Buffer Size"=w430:u32)  [unwired: 6 in]
                n187 = call "Pathhorafech(SubVI)_varios.vi"("Folder path"=path "c:/Trenes", "Nº de acelerómetros"=w402, "Nº inductivos"=w403) -> ("Acel_Paths"=w398:path[])  [unwired: 1 in, 1 out]
                "Nombre de archivo" <- w398
                n188 = Index Array(array=w398) -> (element=w397:path)  [unwired: 1 in]
                n189 = for {
                  tunnel: w398 -> [w439] mode=indexing
                  tunnel: [w438] -> w423 mode=indexing
                  tunnel: [w437] -> w422
                  n190 = Open/Create/Replace File(file path (use dialog)=w439, operation (0:open)=T5."replace or create", access (0:read/write)=enum16{"read/write", "read-only", "write-only"}."read/write", disable buffering (F)=TRUE) -> (refnum out=w438:refnum<file>, error out=w437:errorcluster)  [unwired: 1 in, 2 out]
                }
                n191 = xnode "Invoke Method"("FPGA VI Reference In"=w419, "error in"=w418, "Requested Depth"=w430) -> ("FPGA VI Reference Out"=w432:refnum<k20>, "error out"=w431:errorcluster)  [unwired: 1 out]
                n192 = local read "Report"() -> (w401:string)
                n193 = Path To String(path=w397) -> (string=w395:string)
                n194 = Concatenate Strings("\nFile created: ", w395, "\n", w401) -> (w400:string)
                n195 = xnode "Invoke Method"("FPGA VI Reference In"=w432, "error in"=w431) -> ("FPGA VI Reference Out"=w427:refnum<k20>, "error out"=w426:errorcluster)
                n196 = local write "Report"(w400) -> ()
              }
              frame #1 {
                n197 = while "Data Acquisition" {
                  tunnel: w458 -> [w512]
                  shift-right: [w536] -> _
                  shift-left: u32 0 ("t") -> [w532]
                  tunnel: w456 -> [w537]
                  tunnel: w455 -> [w535]
                  shift-right: [w538] -> w460
                  shift-left: w457 -> [w529]
                  tunnel: [w533] -> w461
                  tunnel: w454 -> [w516]
                  tunnel: [w517] -> w459
                  shift-right: [w515] -> w452
                  shift-left: w453 -> [w525]
                  stop <- w534 stop-if-true
                  # "Detector de presencia"
                  # "Mide el tiempo de paso del tren y con ello se puede calcular\nla velocidad la unidad"
                  n198 = xnode "Invoke Method"("FPGA VI Reference In"=w512, "error in"=w529, "Number of Elements"=w532, "Timeout (ms)"=0) -> ("FPGA VI Reference Out"=w509:refnum<k20>, "error out"=w514:errorcluster, "Data"=w528:fxp<+/-,24,4>[], "Elements Remaining"=w530:u32)
                  n199 = case "Data Ready" shown="Default" w532 {
                    tunnel: w537 -> [w560 _]
                    tunnel: [w559 u32 0 ("t")] -> w536
                    tunnel: w535 -> [w561 _]
                    tunnel: w530 -> [w558 _]
                    tunnel: w528 -> [_ w583]
                    tunnel: w525 -> [w557 w582]
                    tunnel: [w557 w584] -> w515
                    tunnel: w516 -> [w556 w581]
                    tunnel: [w556 w580] -> w517
                    frame 0 {
                      # "En este caso se compara los elementos que quedan\nen la FIFO del controlador con el tamaño dell bloque\nque aparece en el panel frontal. Si el número de \nelementos en la FIFO es mayor o igual que el tamaño\n del bloque se pasa al siguiente caso y se guardan \nlos datos en un archivo. El reloj que aparece es una\nespera para no consumir recursos."
                      n200 = Greater Or Equal?(x=w558, y=w561) -> (x >= y?=w562:bool)
                      n201 = case shown="False" w562 {
                        tunnel: [u32 0 ("Block Size") w566] -> w559
                        tunnel: [w565 0 ("t")] -> w563
                        tunnel: w560 -> [w565 _]
                        tunnel: w561 -> [_ w566]
                        frame False {
                        }
                        frame True {
                        }
                      }
                      n202 = call "WaitMinTimeBetweenCall.vi"("Minimum ms between calls"=w563) -> ()  [unwired: 2 in]
                    }
                    frame Default {
                      n203 = To Single Precision Float(number=w583) -> (single precision float=w570:sgl[])
                      n204 = Decimate 1D Array(w570) -> (w576:sgl[], w579:sgl[], w578:sgl[], w577:sgl[], w575:sgl[], w574:sgl[], w573:sgl[], w572:sgl[], w571:sgl[], w568:sgl[])
                      n205 = Build Array(w576, w579, w578, w577, w575, w574, w573, w572, w571, w568) -> (w569:sgl[][])
                      n206 = for {
                        tunnel: T6."little-endian" ("byte order (0:big-endian, network order)") -> [w593]
                        shift-right: [w587] -> w584
                        shift-left: w582 -> [w588]
                        tunnel: w569 -> [w591] mode=indexing
                        tunnel: w581 -> [w590] mode=indexing
                        tunnel: [w589] -> w580 mode=indexing
                        n207 = Write to Binary File(file (use dialog)=w590, data=w591, error in=w588, 5:FALSE ("prepend array or string size? (T)"), 9:w593) -> (refnum out=w589:refnum<file>, error out=w587:errorcluster)  [unwired: 2 out]
                      }
                    }
                  }
                  n208 = xnode "Read/Write Control"("FPGA VI Reference In"=w509, "error in"=w514) -> ("FPGA VI Reference Out"=w527:refnum<k20>, "error out"=w526:errorcluster, "Parar"=w505:bool, "Nº Ruedas 1"=→"Nº Ruedas 1":i32, "NºRuedas 2"=→"NºRuedas 2":i32)
                  "Parar" <- w505
                  n209 = case shown="False" w505 {
                    tunnel: [w543 w551] -> w506
                    tunnel: [w544 0.0] -> w520
                    frame False {
                      n210 = local read "Inicio pasada"() -> (w547:timestamp)
                      n211 = Get Date/Time In Seconds() -> (seconds since 1Jan1904=w546:timestamp)
                      n212 = local read "Tiempo de adquisicion"() -> (w539:dbl)
                      n213 = To Double Precision Float(number=w546) -> (double precision float=w545:dbl)
                      n214 = To Double Precision Float(number=w547) -> (double precision float=w548:dbl)
                      n215 = Subtract(x=w545, y=w548) -> (x-y=w544:dbl)
                      "Tiempo de paso (s)" <- w544
                      n216 = local write "Tiempo"(w545) -> ()
                      n217 = local read "Boton Adquirir?"() -> (w540:bool)
                      n218 = Greater?(x=w544, y=w539) -> (0:w542:bool)
                      n219 = Select(t=w542, s=w540, f=FALSE) -> (s? t:f=w543:bool)
                    }
                    frame True {
                      n220 = local read "Tiempo"() -> (w555:dbl)
                      n221 = local read "Tiempo extra al detector de paso (s)"() -> (w550:dbl)
                      n222 = Get Date/Time In Seconds() -> (seconds since 1Jan1904=w552:timestamp)
                      n223 = To Double Precision Float(number=w552) -> (double precision float=w553:dbl)
                      n224 = Subtract(x=w553, y=w555) -> (x-y=w554:dbl)
                      n225 = Greater?(x=w554, y=w550) -> (0:w551:bool)
                    }
                  }
                  "Fin" <- w506
                  n226 = local read "Timeout ruedas"() -> (w504:dbl)
                  n227 = xnode ("CheckLate")("FPGA VI Reference In"=w527, "error in"=w526) -> ("FPGA VI Reference Out"=w511:refnum<k20>, "error out"=w522:errorcluster, "Buffer Underflow"=→"Buffer Underflow":bool, "Buffer Overflow"=w513:bool)
                  "Buffer Overflow" <- w513
                  n228 = Greater?(x=w520, y=w504) -> (0:w518:bool)
                  "Timeout ruedas" <- w518
                  n229 = call "ErrorOverFlow.vi"("Buffer Overflow"=w513) -> ("error out"=w521:errorcluster)
                  n230 = Merge Errors(w522, w521) -> (w510:errorcluster)
                  n231 = Unbundle By Name(w515) -> ("status"=w519:bool)
                  n232 = Unbundle By Name(w510) -> ("status"=w524:bool)
                  n233 = Compound Arithmetic op=OR(w524, w506, w518, w519) -> (w534:bool)
                  "result" <- w534
                  n234 = case "Flush" shown="True" w534 {
                    tunnel: [w594 w599] -> w538
                    tunnel: [w595 w598] -> w533
                    tunnel: w511 -> [w595 w597]
                    tunnel: w510 -> [w594 w596]
                    frame False {
                    }
                    frame True {
                      n235 = xnode "Invoke Method"("FPGA VI Reference In"=w597, "error in"=w596) -> ("FPGA VI Reference Out"=w598:refnum<k20>, "error out"=w599:errorcluster)
                    }
                  }
                  "Block Size" <- w535
                  "Time to Acquire Block (ms)" <- w537
                }
                n236 = call <vilib>:"Watchdog Whack.vi"("error in (no error)"=w447, "reset watchdog after expire? (F)"=TRUE, "watchdogID in"=w448) -> ("error out"=w444:errorcluster, "watchdogID out"=w445:u64)  [unwired: 2 in, 1 out]
                n237 = local read "RFID LR6 on?"() -> (w443:bool)
                n238 = case shown="True" w443 {
                  tunnel: w450 -> [w462 w468]
                  tunnel: [w462 w467] -> w449
                  frame False {
                  }
                  frame True {
                    n239 = while {
                      shift-right: [w475] -> w467
                      shift-left: w468 -> [w476]
                      shift-right: [w474] -> w465
                      shift-left: string[] [] -> [w473]
                      shift-right: [w469] -> w463
                      shift-left: i32[] [] -> [w470]
                      i -> [w471]
                      stop <- w472 stop-if-true
                      n240 = case shown="No Error" w476 {
                        selector: w476 -> [w487 _]
                        tunnel: [w486 w502] -> w475
                        tunnel: [w482 string[] []] -> w474
                        tunnel: w473 -> [w481 _]
                        tunnel: w471 -> [w480 _]
                        tunnel: w470 -> [w479 _]
                        tunnel: [w478 i32[] []] -> w469
                        frame No Error {
                          n241 = call "LH6HD.vi"("error in (no error)"=w487, "Action"=enum16{"Init", "Start", "Read", "Stop", "Exit"}."Read") -> ("error out"=w486:errorcluster, "Tag"=w483:string)  [unwired: 8 in]
                          n242 = Not Equal?(x="", y=w483) -> (x != y?=w484:bool)
                          n243 = case shown="False" w484 {
                            tunnel: w483 -> [_ w496]
                            tunnel: [w490 w495] -> w482
                            tunnel: w481 -> [w490 w494]
                            tunnel: w480 -> [_ w491]
                            tunnel: w479 -> [w489 w493]
                            tunnel: [w489 w492] -> w478
                            frame False {
                            }
                            frame True {
                              n244 = Build Array (concatenate)(w494, w496) -> (w495:string[])
                              n245 = Build Array (concatenate)(w493, w491) -> (w492:i32[])
                            }
                          }
                        }
                        frame Error {
                          n246 = local read "LR6 IP address"() -> (w499:string)
                          n247 = local read "DeviceAddress"() -> (w497:u8)
                          n248 = local read "Port LR6"() -> (w500:u16)
                          n249 = call "LH6HD.vi"("DeviceAddress"=w497, "Reader Port"=w500, "IP Address"=w499, "Action"=enum16{"Init", "Start", "Read", "Stop", "Exit"}."Init") -> ("error out"=w502:errorcluster)  [unwired: 6 in, 1 out]
                        }
                      }
                      n250 = Wait Until Next ms Multiple(millisecond multiple=u32 500) -> ()  [unwired: 1 out]
                      n251 = local read "result"() -> (w472:bool)
                      "it-LR6" <- w471
                    }
                    "TAGs LR6" <- w465
                    "it-read-LR6" <- w463
                  }
                }
              }
              frame #2 {
                n252 = local read "RFID LR6 on?"() -> (w621:bool)
                n253 = Array Size(array=w639) -> (size(s)=w637:i32)
                n254 = local read "timeout ms (60000)"() -> (w624:i32)
                n255 = local read "AURA wheel test"() -> (w601:bool)
                n256 = case shown="True" w621 {
                  tunnel: w634 -> [w674 w680]
                  tunnel: [w674 w675] -> w633
                  frame False {
                  }
                  frame True {
                    n257 = call "LH6HD.vi"("error in (no error)"=w680, "Action"=enum16{"Init", "Start", "Read", "Stop", "Exit"}."Stop") -> ("error out"=w675:errorcluster)  [unwired: 8 in, 1 out]
                    n258 = call "Reporting_error.vi"("error out 2"=w675, "Concept"="Active RFID") -> ("Reporting"=w677:string)  [unwired: 1 in]
                    n259 = local read "Report"() -> (w678:string)
                    n260 = Concatenate Strings(w677, w678) -> (w676:string)
                    n261 = local write "Report"(w676) -> ()
                  }
                }
                n262 = local read "bytes to read"() -> (w623:i32)
                n263 = local read "RFID NEM on?"() -> (w622:bool)
                n264 = Decrement(x=w637) -> (x-1=w638:i32)
                n265 = local read "Puerto RFID"() -> (w654:u16)
                n266 = local read "RFID_Error"() -> (w664:errorcluster)
                n267 = local read "IP RFID"() -> (w636:string)
                n268 = local read "RFID_ID"() -> (w663:refnum<k5>)
                n269 = Index Array(array=w639, index=w638) -> (element=w647:refnum<file>)
                n270 = local write "result"(FALSE ("result")) -> ()
                n271 = xnode "Read/Write Control"("FPGA VI Reference In"=w620, "error in"=w619) -> ("FPGA VI Reference Out"=w665:refnum<k20>, "error out"=w616:errorcluster, "Chassis Temperature"=w673:i16)
                n272 = local read "TAGs LR6"() -> (w603:string[])
                n273 = case shown="True" w622 {
                  tunnel: w664 -> [w683 w696]
                  tunnel: w663 -> [w682 w695]
                  tunnel: [w682 w694] -> w662
                  tunnel: [w683 w684] -> w658
                  tunnel: w654 -> [_ w693]
                  tunnel: w636 -> [_ w692]
                  tunnel: [_ w691] -> w618
                  tunnel: w624 -> [_ w690]
                  tunnel: w623 -> [_ w689]
                  frame False {
                  }
                  frame True {
                    n274 = call "RFID_28_03_12.vi"("BYTES TO READ"=w689, "TIMEOUT"=w690, "RFID_Error"=w696, "Puerto RFID"=w693, "IP RFID"=w692, "RFID ID"=w695) -> ("RFID Error"=w684:errorcluster, "connection ID out"=w694:refnum<k5>, "TAGs HEX"=w691:string[])  [unwired: 1 in, 1 out]
                    n275 = call "Reporting_error.vi"("error out 2"=w684, "Concept"="Passive RFID") -> ("Reporting"=w686:string)  [unwired: 1 in]
                    n276 = local read "Report"() -> (w687:string)
                    n277 = Concatenate Strings(w686, w687) -> (w685:string)
                    n278 = local write "Report"(w685) -> ()
                  }
                }
                "TAGs HEX" <- w618
                n279 = Select(t=string[] ["A0000000000000000TESTNEM7", "A0000000000000000TESTNEM8"], s=w601, f=w603) -> (s? t:f=w600:string[])
                n280 = Divide(x=w673, y=4.0) -> (x/y=w612:dbl)
                "Temperatura (ºC)" <- w612
                n281 = local read "Tiempo de paso (s)"() -> (w660:dbl)
                n282 = for {
                  tunnel: w600 -> [w699] mode=indexing
                  tunnel: [w697] -> w627 mode=indexing
                  n283 = Search and Replace String(input string=w699, search string="00") -> (result string=w697:string)  [unwired: 6 in, 3 out]
                }
                n284 = local write "RFID_LR6_Error"(w633) -> ()
                n285 = Index Array(array=w618) -> (element=w632:string)  [unwired: 1 in]
                n286 = local read "Nº Ruedas 1"() -> (w610:i32)
                n287 = local read "NºRuedas 2"() -> (w614:i32)
                n288 = Not Equal?(x=w632, y="" ("delimiter (\\t)")) -> (x != y?=w630:bool)
                "Plataformas?" <- w630
                n289 = Multiply(x=w660, y=1000.0) -> (x*y=w611:dbl)
                n290 = case shown="True" w630 {
                  tunnel: w627 -> [w700 w701]
                  tunnel: [w700 w703] -> w613
                  tunnel: w618 -> [_ w702]
                  frame False {
                  }
                  frame True {
                    n291 = call "Union_TAGs_RFIDs.vi"("TAGs LR6"=w701, "TAGs HEX"=w702) -> ("TAGs"=w703:string[])
                  }
                }
                "TAGs" <- w613
                n292 = local write "RFID_ID"(w662) -> ()
                n293 = local write "RFID_Error"(w658) -> ()
                n294 = Build Array(w612, w611, w610, w614) -> (w615:dbl[])
                n295 = Build Array(w612, w611, w610) -> (w609:dbl[])
                n296 = local read "Direccion 0?"() -> (w608:bool)
                n297 = local read "Nombre de archivo"() -> (w646:path[])
                n298 = for {
                  shift-right: [w709] -> w652
                  shift-left: string[] [] -> [w708]
                  tunnel: w613 -> [w707] mode=indexing
                  n299 = Insert Into Array(array=w708, new element=w707) -> (w709:string[])  [unwired: 1 in]
                }
                n300 = Bundle("error out"=w616, w615, "TAGs"=w613, "Direccion 0?"=w608) -> (w607:T8)  [unwired: 1 in]
                n301 = Delete From Array(array=w646) -> (deleted portion=w645:path)  [unwired: 2 in, 1 out]
                n302 = To Single Precision Float(number=w609) -> (single precision float=w671:sgl[])
                n303 = xnode "Read/Write Control"("FPGA VI Reference In"=w665, "error in"=w616, "Stop"=TRUE ("stop")) -> ("FPGA VI Reference Out"=w649:refnum<k20>, "error out"=w648:errorcluster)
                n304 = call "Reporting_acqu.vi"("output cluster"=w607, "address repoting"=path "C:/Reporting/Reporting_adqu.txt" ("file (use dialog)")) -> ("Reporting"=w604:string)  [unwired: 1 in]
                n305 = Path To String(path=w645) -> (string=w651:string)
                n306 = local read "Report"() -> (w605:string)
                n307 = Write to Binary File(file (use dialog)=w647, data=w671, error in=w668, 5:FALSE ("prepend array or string size? (T)"), 9:T6."little-endian" ("byte order (0:big-endian, network order)")) -> (error out=w644:errorcluster)  [unwired: 3 out]
                n308 = local read "Timeout ruedas"() -> (w661:bool)
                n309 = Build Array (concatenate)(w651, w652) -> (w628:string[])
                n310 = local read "TAGS leidos"() -> (w640:path)
                n311 = Concatenate Strings(w604, w605) -> (w606:string)
                n312 = for {
                  shift-right: [w706] -> w655
                  shift-left: w644 -> [w705]
                  tunnel: w639 -> [w704] mode=indexing
                  n313 = Close File(refnum=w704, error in=w705) -> (error out=w706:errorcluster)  [unwired: 1 out]
                }
                n314 = local write "Report"(w606) -> ()
                n315 = xnode "Invoke Method"("FPGA VI Reference In"=w649, "error in"=w648) -> ("FPGA VI Reference Out"=w657:refnum<k20>, "error out"=w656:errorcluster)
                n316 = call-poly <vilib>:"Write Delimited Spreadsheet.vi"("file path (dialog if empty)"=w640, "1D data"=w628, "append to file? (new file:F)"=TRUE ("transpose? (no:F)"), "transpose? (no:F)"=TRUE ("append to file? (new file:F)"), "delimiter (\\t)"=";" ("delimiter (\\t)")) -> ()  [unwired: 9 in, 2 out]
                n317 = Select(t="TEST", s=w661, f="Procesado") -> (s? t:f=w666:string)
              }
            }
            n318 = call <vilib>:"Watchdog Clear.vi"("error in (no error)"=w356, "watchdogID in"=w357) -> ("error out"=w358:errorcluster)  [unwired: 5 in]
            n319 = Unbundle By Name(w383) -> ("status"=w372:bool)
            n320 = Unbundle By Name(w381) -> ("status"=w373:bool)
            n321 = Merge Errors(w381, w358) -> (w380:errorcluster)
            n322 = Compound Arithmetic op=OR(w372, w373) -> (w370:bool)
            n323 = Select(t="TEST", s=w370, f=w371) -> (s? t:f=w368:string)
          }
          frame "Procesado" {
            n324 = flat-sequence {
              tunnel: w715 -> [w734]
              tunnel: [w734] -> w714
              tunnel: w713 -> [w730]
              tunnel: [w730] -> w712
              frame #0 {
                n325 = local read "Report"() -> (w731:string)
                n326 = call "Reporting_datetime.vi"() -> ("String"=w729:string)  [unwired: 11 in]
                n327 = Concatenate Strings(w729, "\nSTATUS: PROCESSING\nProcessing the measurement\n\n", w731) -> (w733:string)
                n328 = local write "Report"(w733) -> ()
              }
            }
            n329 = local read "Watchdog config"() -> (w721:T1)
            n330 = call <vilib>:"Watchdog Configure.vi"("error in (no error)"=w724, "expiration actions"=w721, "timeout (1 sec)"=300.0) -> ("error out"=w723:errorcluster, "watchdogID"=w720:u64)  [unwired: 1 in, 2 out]
            n331 = flat-sequence {
              tunnel: w723 -> [w741]
              tunnel: w720 -> [w737]
              tunnel: [w736] -> w719
              tunnel: [w735] -> w718
              tunnel: [w952] -> w717
              tunnel: w719 -> [w952]
              tunnel: [w951] -> w716
              tunnel: w718 -> [w951]
              frame #0 {
                n332 = flat-sequence {
                  tunnel: [w813] -> w743
                  tunnel: [w799] -> w742
                  tunnel: w741 -> [w780]
                  tunnel: [w762] -> w738
                  tunnel: [w801] -> w740
                  tunnel: [w753] -> w739
                  tunnel: w737 -> [w781]
                  tunnel: [w778] -> w736
                  tunnel: [w777] -> w735
                  frame #0 {
                    n333 = local read "AURA wheel test"() -> (w751:bool)
                    n334 = case shown="True" w751 {
                      tunnel: [w816 w817] -> w750
                      tunnel: [w815 path[] [path "c:/Trenes_prueba/A_0_TEST.bin", path "c:/Trenes_prueba/A_1_TEST.bin", path "c:/Trenes_prueba/A_2_TEST.bin", path "c:/Trenes_prueba/A_3_TEST.bin", path "c:/Trenes_prueba/A_4_TEST.bin", path "c:/Trenes_prueba/A_5_TEST.bin", path "c:/Trenes_prueba/A_6_TEST.bin", path "c:/Trenes_prueba/A_7_TEST.bin", path "c:/Trenes_prueba/I_0_TEST.bin", path "c:/Trenes_prueba/I_1_TEST.bin"]] -> w749
                      frame False {
                        n335 = local read "Nombre de archivo"() -> (w815:path[])
                        n336 = local read "TAGs"() -> (w816:string[])
                      }
                      frame True {
                        w817 = string[] ["A0000000000000000TESTNEM7", "A0000000000000000TESTNEM8"]
                        n337 = local write "TAGs LR6"(w817) -> ()
                      }
                    }
                    n338 = local read "Tabla_flota"() -> (w798:string[][])
                    n339 = call <vilib>:"Watchdog Whack.vi"("error in (no error)"=w780, "reset watchdog after expire? (F)"=TRUE, "watchdogID in"=w781) -> ("error out"=w777:errorcluster, "watchdogID out"=w778:u64)  [unwired: 2 in, 1 out]
                    n340 = local read "Puntos medios de las ventanas"() -> (w800:dbl[][])
                    n341 = call "Series_ejes_flota.vi"("Tabla_flota"=w798, "Tags"=w750) -> ("Nº Ejes"=w775:i32[], "Series del convoy"=w792:string[])  [unwired: 2 in, 1 out]
                    "Nº Ejes" <- w775
                    n342 = Array Size(array=w749) -> (size(s)=w807:i32)
                    n343 = Add Array Elements(numeric array=w775) -> (sum=w761:i32)
                    "Ejes_convoy" <- w761
                    n344 = Subtract(x=w807, y=2 ("length")) -> (x-y=w809:i32)
                    n345 = Array Size(array=w792) -> (size(s)=→"Nº UTs":i32)
                    n346 = local read "Series_flota"() -> (w797:string[])
                    n347 = Delete From Array(array=w749, length=2, index=w809) -> (deleted portion=w782:path[], array with subset deleted=w801:path[])
                    n348 = Index Array(array=w782) -> (element #2=w776:path)  [unwired: 2 in, 1 out]
                    n349 = call "Distancias_ejes_convoy.vi"("Series_flota1"=w792, "Ejes_UT"=w775, "Puntos medios de las ventanas"=w800, "Series_flota"=w797) -> ("Distancias_entre_ejes_convoy"=w799:dbl[])  [unwired: 1 in]
                    n350 = Read from Binary File(5:sgl 0.0, 9:T6."little-endian" ("byte order (0:big-endian, network order)"), 10:-1 ("count (1)"), 11:w776) -> (0:w805:errorcluster, 2:w784:sgl[], 3:w806:refnum<file>)  [unwired: 1 in, 2 out]
                    n351 = local read "Frecuencia de muestreo (Hz)"() -> (w766:dbl)
                    n352 = local read "Offset_rueda WS 2"() -> (w767:fxp<+/-,24,-4>)
                    n353 = local read "it-LR6"() -> (w787:i32)
                    n354 = local read "it-read-LR6"() -> (w788:i32[])
                    n355 = local read "Plataformas?"() -> (w786:bool)
                    n356 = local read "TAGs"() -> (w790:string[])
                    n357 = local read "TAGs LR6"() -> (w789:string[])
                    n358 = Close File(refnum=w806, error in=w805) -> (error out=w745:errorcluster)  [unwired: 1 out]
                    n359 = Array Size(array=w784) -> (size(s)=w796:i32)
                    n360 = Subtract(x=w796, y=3 ("length")) -> (x-y=w794:i32)
                    n361 = Delete From Array(array=w784, length=3, index=w794) -> (array with subset deleted=w773:sgl[])  [unwired: 1 out]
                    n362 = call "TAGs_AURAwheel.vi"("Nº Ejes"=w775, "TAGs"=w790, "Ejes_convoy"=w761, "it-LR6"=w787, "TAGs LR6"=w789, "it-read-LR6"=w788, "Plataformas?"=w786) -> ("TAGS_AURA"=→"TAGs_AURAwheel":string[][])  [unwired: 1 in]
                    n363 = call "Analogico_digital.vi"("Array"=w773, "Offset WS"=w767, "Frecuencia muestreo"=w766) -> ("array w/ subset deleted"=w768:sgl[], "Tiempo\npaso"=w765:dbl)  [unwired: 6 in]
                    n364 = call "Puntos medio de pulso.vi"("DI Inductivo"=w768) -> ("Puntos"=w813:sgl[], "Número de ejes"=w755:i32)  [unwired: 1 in]
                    "Número de ejes detectados" <- w755
                    n365 = disable-structure shown="Disabled" {
                      disable-tunnel: w773 -> [w825 w828]
                      disable-tunnel: [FALSE ("element") TRUE ("element")] -> w770
                      disable-tunnel: [w819 w827] -> w769
                      frame Disabled {
                        n366 = Equal?(x=w825, y=0.0) -> (x = y?=w822:bool[])
                        n367 = Equal?(x=w825, y=1.0) -> (x = y?=w823:bool[])
                        n368 = Or(x=w822, y=w823) -> (x .or. y?=w819:bool[])
                      }
                      frame Enabled {
                        n369 = Greater?(x=w828, y=0.1) -> (0:w827:bool[])
                      }
                    }
                    n370 = Decrement(x=w755) -> (x-1=w812:i32)
                    n371 = call "Reporting_error.vi"("error out 2"=w745, "Concept"="Measurement reading") -> ("Reporting"=w747:string)  [unwired: 1 in]
                    n372 = Get Volume Info(11:path "c:/" ("path")) -> (1:w756:i64)  [unwired: 1 in, 5 out]
                    "Disco Duro Disponible (bytes)" <- w756
                    n373 = local read "Report"() -> (w748:string)
                    n374 = call "Calculo_Velocidad.vi"("Tiempo de paso (s)"=w765, "Ejes"=w812, "Puntos iniciales de las ventanas"=w799) -> ("V (m/s)"=→"V (m/s)":dbl, "Longitud de la unidad"=→"Longitud de la unidad":dbl)
                    n375 = Concatenate Strings(w747, w748) -> (w746:string)
                    n376 = Equal?(x=w761, y=w755) -> (x = y?=w753:bool)
                    n377 = Not Equal?(x=w755, y=0) -> (x != y?=w752:bool)
                    n378 = Search 1D Array(1D array=w769, element=w770) -> (index of element=w771:i32)  [unwired: 1 in]
                    n379 = local write "Report"(w746) -> ()
                    n380 = Build Array(w761, w755, w756) -> (w760:i64[])
                    n381 = Equal?(x=w771, y=-1) -> (x = y?=w774:bool)
                    n382 = Compound Arithmetic op=AND(w753, w752, w774) -> (w762:bool)
                    "Archivo\nvalido?" <- w762
                    n383 = Bundle(w760, w762) -> (w758:cluster{i64[], bool})  [unwired: 1 in]
                    n384 = call "Reporting_proc.vi"("output cluster 2"=w758, "address repoting"=path "C:/Reporting/Reporting_proc.txt" ("file (use dialog)")) -> ("Reporting"=w757:string)  [unwired: 1 in]
                    n385 = local read "Report"() -> (w763:string)
                    n386 = Concatenate Strings(w757, w763) -> (w764:string)
                    n387 = local write "Report"(w764) -> ()
                  }
                }
                n388 = case shown="True" w738 {
                  tunnel: w743 -> [_ w863]
                  tunnel: w742 -> [_ w861]
                  tunnel: w740 -> [_ w862]
                  tunnel: w739 -> [w830 _]
                  frame False {
                    n389 = local read "Nombre de archivo"() -> (w831:path[])
                    n390 = for {
                      tunnel: w831 -> [w833] mode=indexing
                      tunnel: w830 -> [w832]
                      n391 = flat-sequence {
                        tunnel: w833 -> [w843]
                        tunnel: [w843] -> w836
                        tunnel: [w842] -> w835
                        tunnel: w832 -> [w841]
                        tunnel: w836 -> [w850]
                        tunnel: [w849] -> w834
                        tunnel: w835 -> [w849]
                        tunnel: w834 -> [w852]
                        frame #0 {
                          w842 = path "c:/Est_Adq.csv" ("file path (use dialog)")
                          n392 = Path To String(path=w843) -> (string=w844:string)
                          n393 = Select(t="Nº Ejes detectados WS diferente a Nº Ejes TAGs" ("delimiter (\\t)"), s=w841, f="La señal del inductivo no es digital" ("delimiter (\\t)")) -> (s? t:f=w838:string)
                          n394 = Build Array(w844, w838) -> (w837:string[])
                          n395 = call-poly <vilib>:"Write Delimited Spreadsheet.vi"("file path (dialog if empty)"=w842, "1D data"=w837, "append to file? (new file:F)"=FALSE ("transpose? (no:F)"), "transpose? (no:F)"=TRUE ("append to file? (new file:F)"), "delimiter (\\t)"=";" ("delimiter (\\t)")) -> ()  [unwired: 9 in, 2 out]
                        }
                        frame #1 {
                          n396 = local read "Borrar archivos\nadquisicion con error"() -> (w848:bool)
                          n397 = case shown="True" w848 {
                            tunnel: w850 -> [_ w851]
                            frame False {
                            }
                            frame True {
                              n398 = Delete(path (use dialog)=w851) -> ()  [unwired: 1 in, 6 out]
                            }
                          }
                        }
                        frame #2 {
                          n399 = File/Directory Info(path=w852) -> (size=w855:i64)  [unwired: 1 in, 6 out]
                          n400 = Greater?(x=w855, y=i64 1000000) -> (0:w853:bool)
                          n401 = case shown="True" w853 {
                            tunnel: w852 -> [_ w856]
                            frame False {
                            }
                            frame True {
                              n402 = Delete(path (use dialog)=w856) -> ()  [unwired: 4 in, 3 out]
                            }
                          }
                        }
                      }
                    }
                  }
                  frame True {
                    n403 = flat-sequence {
                      tunnel: w863 -> [w940]
                      tunnel: w862 -> [w937]
                      tunnel: w861 -> [w941]
                      tunnel: [w924] -> w860
                      frame #0 {
                        # "SALIDA \n\nMáximos por rueda inductivo"
                        # "8 acelerómetros"
                        # "Velocidad"
                        n404 = local read "Frecuencia de muestreo (Hz)"() -> (w939:dbl)
                        n405 = local read "Distancia de acelerómetros"() -> (w929:dbl[])
                        n406 = local read "Parámetros acelerómetros"() -> (w936:dbl[])
                        n407 = local read "Número de ejes detectados"() -> (w935:i32)
                        n408 = local read "Distancias generales"() -> (w934:dbl[])
                        n409 = local read "dt RMS"() -> (w938:dbl)
                        n410 = local read "Direccion 0?"() -> (w926:bool)
                        n411 = Index Array(array=w934, index=1) -> (element=w932:dbl)
                        n412 = Select(t=0.0, s=w926, f=w932) -> (s? t:f=w930:dbl)
                        n413 = Subtract(x=w930, y=w929) -> (x-y=w928:dbl[])
                        n414 = Absolute Value(x=w928) -> (abs(x)=w927:dbl[])
                        n415 = call "Procesado_aRMS_BIdirecc.vi"("Paths_canales_aRMS"=w937, "Ejes Procesados"=w935, "Distancias\nacelerometros"=w927, "Distancias generales (m)"=w934, "Distancias centrales de las ruedas\n               configuración (m)"=w941, "Frecuencia de muestreo"=w939, "Parámetros acelerómetros"=w936, "dt RMS 2"=w938, "Puntos"=w940) -> ("Max RMS Ruedas"=w925:dbl[][])  [unwired: 2 in]
                        n416 = Transpose 2D Array(2D array=w925) -> (transposed array=w924:dbl[][])
                        "Max RMS Ruedas" <- w924
                        n417 = call "Reporting_proc_RMS.vi"("Max RMS Ruedas"=w924) -> ("String"=w922:string)
                        n418 = local read "Report"() -> (w923:string)
                        n419 = Concatenate Strings(w922, w923) -> (w921:string)
                        n420 = local write "Report"(w921) -> ()
                      }
                    }
                    n421 = local read "Use Aura?"() -> (w859:bool)
                    n422 = local read "TAGs_AURAwheel"() -> (w858:string[][])
                    n423 = local read "Nº Ejes"() -> (w857:i32[])
                    n424 = for {
                      tunnel: w859 -> [w867]
                      tunnel: w858 -> [w866] mode=indexing
                      shift-right: [w865] -> _
                      shift-left: w860 -> [w868]
                      tunnel: w857 -> [w864] mode=indexing
                      # "dev.api.aurawheel.com"
                      n425 = case shown="True" w867 {
                        tunnel: w868 -> [w869 w888]
                        tunnel: w866 -> [_ w889]
                        tunnel: [w869 w887] -> w865
                        tunnel: w864 -> [_ w885]
                        frame False {
                        }
                        frame True {
                          w873 = "\n"
                          w896 = cluster{"status":string} {"status"=""}
                          n426 = local read "Parametros AuraWheel"() -> (w920:string[])
                          n427 = Delete From Array(array=w888, length=w885, index (row)=0) -> (deleted portion=w884:dbl[][], array with subset deleted=w887:dbl[][])  [unwired: 1 in]
                          n428 = Get Date/Time In Seconds() -> (seconds since 1Jan1904=w917:timestamp)
                          n429 = Format Date/Time String(time format string (%c)="%H:%M:%S%3u", seconds (now)=w917) -> (date/time string=w915:string)  [unwired: 1 in]
                          n430 = Get Date/Time In Seconds() -> (seconds since 1Jan1904=w892:timestamp)
                          n431 = Scan From String(format string="%d:%d:%f", input string=w915) -> (output 1=w912:i32, output 2=w911:i32, output 3=w909:dbl)  [unwired: 5 in, 3 out]
                          n432 = local read "V (m/s)"() -> (w880:dbl)
                          n433 = local read "Temperatura (ºC)"() -> (w890:dbl)
                          n434 = Multiply(x=w880, y=3.6) -> (x*y=w878:dbl)
                          n435 = Multiply(x=w909, y=1000.0) -> (x*y=w905:dbl)
                          n436 = call "Time_to_ms.vi"("seconds since 1Jan1904"=w892) -> ("Numeric"=w891:dbl)  [unwired: 1 in]
                          n437 = Multiply(x=w911, y=60000) -> (x*y=w906:i32)
                          n438 = Multiply(x=3600000, y=w912) -> (x*y=w907:i32)
                          n439 = Index Array(array=w920) -> (element #1=w883:string, element #2=w882:string, element #3=w881:string)  [unwired: 3 in]
                          n440 = call "aw_WRDCluster_8acel.vi"("Array TAGs"=w889, "Max RMS Ruedas"=w884, "TimeStamp"=w891, "p_sp"=w878, "p_tp"=w890) -> ("JSON cluster"=w918:T9)  [unwired: 1 in]
                          n441 = Compound Arithmetic op=ADD(w907, w906, w905) -> (w904:dbl)
                          n442 = To Variant(anything=w918) -> (Variant=w901:variant)
                          n443 = To Unsigned Long Integer(number=w904) -> (unsigned 32bit integer=w903:u32)
                          n444 = call "gjson_Create.vi"("JSON Object in"=w901) -> ("error out"=w899:errorcluster, "JSON String Out"=w900:string)  [unwired: 9 in]
                          n445 = Number To Decimal String(number=w903) -> (decimal integer string=w902:string)  [unwired: 1 in]
                          n446 = To Variant(anything=w896) -> (Variant=w895:variant)
                          n447 = call "aw_SendData.vi"("pwd"=w883, "x-nem-datetime"=w902, "User"=w882, "error in"=w899, "JSON Object"=w900, "URL"=w881) -> ("error out"=w897:errorcluster, "Response JSON"=w898:string, "Response headers"=w874:string)  [unwired: 3 in]
                          "Response headers" <- w874
                          n448 = call "gjson_Parse.vi"("error in"=w897, "JSON String In"=w898, "JSON Cluster"=w895) -> ("error out"=w893:errorcluster, "JSON Cluster Out"=w894:variant)  [unwired: 7 in]
                          n449 = Variant To Data(error in=w893, type=w896, Variant=w894) -> (data=→"data":cluster{"status":string}, error out=w875:errorcluster)
                          "error AURA" <- w875
                          n450 = local read "Report"() -> (w871:string)
                          n451 = call "Reporting_error.vi"("error out 2"=w875, "Concept"="A.U.R.A. Wheel Connection") -> ("Reporting"=w876:string)  [unwired: 1 in]
                          n452 = Concatenate Strings(w876, w873, w873, w874, w873) -> (w872:string)
                          "Report_AURA" <- w872
                          n453 = Concatenate Strings(w872, w871) -> (w870:string)
                          n454 = local write "Report"(w870) -> ()
                        }
                      }
                    }
                  }
                }
              }
              frame #1 {
                n455 = local read "Archivo\nvalido?"() -> (w948:bool)
                n456 = local read "Bytes libre despues de borrar"() -> (w949:u32)
                n457 = local read "Report_AURA"() -> (w945:string)
                n458 = local read "Max archivos"() -> (w946:u32)
                n459 = local read "Path LOG"() -> (w947:path)
                n460 = local read "LOG.txt"() -> (w942:path)
                n461 = local read "Report"() -> (w944:string)
                n462 = local read "Bytes min libre"() -> (w950:u32)
                n463 = local read "TAGS leidos"() -> (w953:path)
                n464 = File/Directory Info(path=w953) -> (size=w956:i64)  [unwired: 1 in, 6 out]
                n465 = case shown="True" w948 {
                  frame False {
                  }
                  frame True {
                    n466 = local read "Nombre de archivo"() -> (w958:path[])
                    n467 = call "Comprimir_a_1_archivo.vi"("Acel_paths"=w958) -> ("path_Pasada"=→"created path":path)
                  }
                }
                n468 = Greater?(x=w956, y=i64 1000000) -> (0:w954:bool)
                n469 = case shown="True" w954 {
                  tunnel: w953 -> [_ w959]
                  frame False {
                  }
                  frame True {
                    n470 = Delete(path (use dialog)=w959) -> ()  [unwired: 4 in, 3 out]
                  }
                }
                n471 = call "BORRADO_MEJORADO_Gonzalo.vi"("Bytes LIBRE OK"=w949, "Bytes Minimo de Memoria libre"=w950) -> ()  [unwired: 10 in]
                n472 = call "Saving_LOG.vi"("Path"=w942, "Report"=w944, "Report AURA"=w945, "Path Carpeta"=w947, "Nº Archivos Max"=w946) -> ("Report"=w943:string)  [unwired: 9 in, 1 out]
                n473 = local write "Report"(w943) -> ()
              }
            }
            n474 = call <vilib>:"Watchdog Clear.vi"("error in (no error)"=w716, "watchdogID in"=w717) -> ("error out"=w710:errorcluster)  [unwired: 5 in]
            n475 = Merge Errors(w712, w710) -> (w728:errorcluster)
            n476 = Unbundle By Name(w728) -> ("status"=w726:bool)
            n477 = Select(t="TEST", s=w726, f="Espera") -> (s? t:f=w725:string)
          }
          frame "TEST" {
            n478 = flat-sequence {
              tunnel: [w975] -> w962
              tunnel: w964 -> [w975]
              frame #0 {
                n479 = call "Reporting_datetime.vi"() -> ("String"=w974:string)  [unwired: 11 in]
                n480 = local read "Report"() -> (w976:string)
                n481 = Concatenate Strings(w974, "\nSTATUS: ERROR TEST\n\n", w976) -> (w978:string)
                n482 = local write "Report"(w978) -> ()
              }
            }
            n483 = local read "Watchdog config"() -> (w969:T1)
            n484 = call <vilib>:"Watchdog Configure.vi"("error in (no error)"=w960, "expiration actions"=w969, "timeout (1 sec)"=200.0) -> ("error out"=w970:errorcluster, "watchdogID"=w967:u64)  [unwired: 1 in, 2 out]
            n485 = Merge Errors(w962, w960) -> (w961:errorcluster)
            n486 = flat-sequence {
              tunnel: [w988] -> w973
              tunnel: w970 -> [w983]
              tunnel: w961 -> [w1001]
              tunnel: [w984] -> w971
              tunnel: w967 -> [w982]
              tunnel: [w981] -> w966
              tunnel: [w980] -> w965
              frame #0 {
                n487 = call <vilib>:"Watchdog Whack.vi"("error in (no error)"=w983, "reset watchdog after expire? (F)"=TRUE, "watchdogID in"=w982) -> ("error out"=w980:errorcluster, "watchdogID out"=w981:u64)  [unwired: 2 in, 1 out]
                n488 = Get Date/Time In Seconds() -> (seconds since 1Jan1904=w995:timestamp)
                n489 = local read "Ultimo TEST"() -> (w996:timestamp)
                n490 = To Double Precision Float(number=w995) -> (double precision float=w997:dbl)
                n491 = Subtract(x=w997, y=3600.0) -> (x-y=w999:dbl)
                n492 = To Time Stamp(1:w999) -> (0:w1000:timestamp)
                n493 = In Range and Coerce(upper limit=w995, x=w996, lower limit=w1000) -> (In Range?=w994:bool)  [unwired: 1 out]
                n494 = case shown="False" w994 {
                  tunnel: w1001 -> [w1011 w1035]
                  tunnel: [w1011 w1035] -> w984
                  frame False {
                    n495 = local read "Timeout ruedas"() -> (w1012:bool)
                    n496 = local read "Aviso no detección"() -> (w1015:string)
                    n497 = local read "Aviso temperatura"() -> (w1014:string)
                    n498 = case shown="True" w1012 {
                      selector: w1012 -> [_ w1032]
                      tunnel: ["\r" w1033] -> w1010
                      frame False {
                      }
                      frame True {
                        w1022 = "\n"
                        n499 = local read "Nº Ruedas 1"() -> (w1029:i32)
                        n500 = local read "NºRuedas 2"() -> (w1024:i32)
                        n501 = call "ErrorRuedas.vi"("Buffer Overflow"=w1032) -> ("error out"=w1034:errorcluster)
                        n502 = Number To Decimal String(number=w1029) -> (decimal integer string=w1027:string)  [unwired: 1 in]
                        n503 = Number To Decimal String(number=w1024) -> (decimal integer string=w1023:string)  [unwired: 1 in]
                        n504 = Concatenate Strings("Error Wheel sensors", "\n", "WS1 (wheels):", w1027, w1022, "WS2 (wheels):", w1023, w1022) -> (w1025:string)
                        n505 = call "Error.vi"("Error con..."=w1025, "error comunicacion 2"=w1034) -> ("String"=w1033:string)
                      }
                    }
                    n506 = local read "DC OK"() -> (w1013:string)
                    n507 = call "Cabecera.vi"() -> ("String"=w1020:string)
                    n508 = call "Adquisicion.vi"("Aviso no detección"=w1015) -> ("String"=w1019:string)
                    n509 = call "Temperatura.vi"("Aviso temperatura"=w1014) -> ("String"=w1018:string)
                    n510 = call "Fuente.vi"("DC OK"=w1013) -> ("String"=w1017:string)
                    n511 = call "FPGA.vi"("error out"=w1011) -> ("String"=w1016:string)
                    n512 = Concatenate Strings(w1020, w1019, w1018, w1017, w1016, w1010) -> (w1003:string)
                    n513 = local read "Report"() -> (w1002:string)
                    n514 = Get Date/Time In Seconds() -> ()  [unwired: 1 out]
                    n515 = Concatenate Strings(w1003, w1002) -> (w1005:string)
                    n516 = local read "Max archivos"() -> (w1006:u32)
                    n517 = local read "Path LOG"() -> (w1009:path)
                    n518 = local read "LOG.txt"() -> (w1007:path)
                    n519 = call "Saving_LOG.vi"("Path"=w1007, "Report"=w1005, "Report AURA"=w1003, "Path Carpeta"=w1009, "Nº Archivos Max"=w1006) -> ("Report"=w1008:string)  [unwired: 9 in, 1 out]
                    n520 = local write "Report"(w1008) -> ()
                    "Ultimo TEST" <- timestamp(3608692059.513 s since 1904-01-01) ("Ultimo TEST")
                  }
                  frame True {
                  }
                }
                n521 = local read "Fallo fotocelula"() -> (w987:bool)
                n522 = Unbundle By Name(w984) -> ("status"=w985:bool)
                n523 = local read "T fuera rango"() -> (w993:bool)
                n524 = Compound Arithmetic op=OR(w985, w987) -> (w986:bool)
                n525 = local write "Reset del controlador"(w986) -> ()
                n526 = Select(t="Escape", s=w993, f="Espera") -> (s? t:f=w990:string)
                n527 = Select(t="Configuracion", s=w986, f=w990) -> (s? t:f=w988:string)
              }
            }
            n528 = call <vilib>:"Watchdog Clear.vi"("error in (no error)"=w965, "watchdogID in"=w966) -> ("error out"=w963:errorcluster)  [unwired: 5 in]
          }
          frame "Calibracion" {
            n529 = flat-sequence {
              tunnel: w1051 -> [w1235]
              tunnel: w1050 -> [w1234]
              tunnel: [w1235] -> w1049
              tunnel: [w1234] -> w1048
              frame #0 {
                n530 = local read "Report"() -> (w1231:string)
                n531 = call "Reporting_datetime.vi"() -> ("String"=w1230:string)  [unwired: 11 in]
                n532 = Concatenate Strings(w1230, "\nSTATUS: CALIBRATION\n\n\n", w1231) -> (w1233:string)
                n533 = local write "Report"(w1233) -> ()
              }
            }
            n534 = flat-sequence {
              tunnel: w1048 -> [w1055]
              tunnel: w1049 -> [w1056]
              tunnel: [w1056] -> w1044
              tunnel: [w1055] -> w1043
              tunnel: [w1053] -> w1042
              tunnel: w1044 -> [w1061]
              tunnel: w1043 -> [w1060]
              tunnel: w1042 -> [w1057]
              tunnel: [w1059] -> w1041
              tunnel: [w1058] -> w1040
              tunnel: w1041 -> [w1173]
              tunnel: w1040 -> [w1172]
              tunnel: [w1173] -> w1039
              tunnel: [w1172] -> w1038
              tunnel: [w1156] -> w1037
              tunnel: [w1155] -> w1036
              tunnel: [w1216] -> w1045
              tunnel: [w1217] -> w1046
              tunnel: w1039 -> [w1217]
              tunnel: w1038 -> [w1216]
              tunnel: w1037 -> [w1215]
              tunnel: w1036 -> [w1211]
              frame #0 {
                n535 = call "Folder_creation_calibration.vi"() -> ("path"=w1054:path, "date/time string"=w1053:string, "calibration log"=→"calibration log":path)  [unwired: 2 in]
                "Folder" <- w1054
                n536 = Create Folder(path (use dialog)=w1054) -> ()  [unwired: 2 in, 3 out]
              }
              frame #1 {
                n537 = for {
                  N: 11 -> [_]
                  shift-right: [w1086] -> w1059
                  shift-left: w1061 -> [w1085]
                  shift-right: [w1087] -> w1058
                  shift-left: w1060 -> [w1084]
                  tunnel: w1057 -> [w1063]
                  i -> [w1079]
                  n538 = xnode "Invoke Method"("FPGA VI Reference In"=w1085, "error in"=w1084) -> ("FPGA VI Reference Out"=w1083:refnum<k20>, "error out"=w1081:errorcluster)  [unwired: 1 in]
                  n539 = Increment(x=w1079) -> (x+1=w1078:i32)
                  n540 = Number To Decimal String(number=w1078) -> (decimal integer string=w1077:string)  [unwired: 1 in]
                  n541 = flat-sequence {
                    tunnel: w1083 -> [w1151]
                    tunnel: [w1151] -> w1082
                    tunnel: w1081 -> [w1150]
                    tunnel: [w1150] -> w1080
                    tunnel: w1077 -> [w1149]
                    frame #0 {
                      n542 = local read "Report"() -> (w1146:string)
                      n543 = Concatenate Strings("\nAcquiring file: ", w1149, "/11\n" ("string"), w1146) -> (w1145:string)
                      n544 = local write "Report"(w1145) -> ()
                    }
                  }
                  n545 = flat-sequence {
                    tunnel: w1080 -> [w1090]
                    tunnel: w1082 -> [w1091]
                    tunnel: [w1091] -> w1076
                    tunnel: [w1090] -> w1075
                    tunnel: [w1088] -> w1064
                    tunnel: w1063 -> [w1088]
                    tunnel: [w1105] -> w1074
                    tunnel: [w1104] -> w1073
                    tunnel: [w1103] -> w1072
                    tunnel: [w1102] -> w1071
                    tunnel: [w1101] -> w1070
                    tunnel: [w1100] -> w1069
                    tunnel: w1076 -> [w1108]
                    tunnel: w1075 -> [w1107]
                    tunnel: w1064 -> [w1092]
                    tunnel: [w1131] -> w1068
                    tunnel: [w1116] -> w1067
                    tunnel: [w1130] -> w1066
                    tunnel: [w1115] -> w1065
                    tunnel: w1074 -> [w1129]
                    tunnel: w1073 -> [w1128]
                    tunnel: w1072 -> [w1127]
                    tunnel: w1071 -> [w1126]
                    tunnel: w1070 -> [w1125]
                    tunnel: w1069 -> [w1124]
                    tunnel: w1068 -> [w1141]
                    tunnel: w1067 -> [w1140]
                    tunnel: w1066 -> [w1142]
                    tunnel: w1065 -> [w1132]
                    tunnel: [w1143] -> w1087
                    tunnel: [w1144] -> w1086
                    frame #0 {
                      n546 = Wait (ms)(milliseconds to wait=u32 1000) -> ()  [unwired: 1 out]
                    }
                    frame #1 {
                      n547 = local read "Frecuencia de muestreo y módulo CRIO"() -> (w1109:T2)
                      n548 = local read "Escaneos de la FIFO por canal"() -> (w1112:u32)
                      n549 = local read "Frecuencia de muestreo (Hz)"() -> (w1111:dbl)
                      n550 = local read "Nº de acelerómetros"() -> (w1114:i32)
                      n551 = local read "Nº inductivos"() -> (w1113:i32)
                      n552 = local read "Count(mSec)"() -> (w1110:u32)
                      n553 = Get Date/Time In Seconds() -> (seconds since 1Jan1904=→"Inicio pasada 2":timestamp)
                      n554 = Bundle("Frecuencia de muestreo y módulo CRIO"=w1109, "Count(mSec)"=w1110, "Frecuencia de muestreo (Hz)"=w1111, "Escaneos de la FIFO por canal"=w1112, "Nº inductivos"=w1113, "Nº de acelerómetros"=w1114) -> (w1106:T10)  [unwired: 1 in]
                      n555 = call "Config_calibr.vi"("error in (no error)"=w1107, "Date Folder"=w1092, "Acq parameters"=w1106, "Refnum in"=w1108) -> ("error out"=w1104:errorcluster, "Block Size"=w1102:u32, "Time to Acquire Block (ms)"=w1103:i32, "Refnum out"=w1105:refnum<k20>, "refnum out"=w1101:refnum<file>, "path"=w1094:path, "error out 2"=w1100:errorcluster)  [unwired: 1 in]
                      "path calib" <- w1094
                      n556 = Path To String(path=w1094) -> (string=w1095:string)
                      n557 = local read "Report"() -> (w1099:string)
                      n558 = Concatenate Strings("\nFile created: ", w1095, "\n", w1099) -> (w1098:string)
                      n559 = local write "Report"(w1098) -> ()
                    }
                    frame #2 {
                      n560 = local read "Inicio pasada 2"() -> (w1123:timestamp)
                      n561 = call "Acq_calibr.vi"("Refnum in"=w1129, "refnum in"=w1125, "Time to Acquire Block (ms)"=w1127, "Block Size"=w1126, "error out 3"=w1124, "error in (no error)"=w1128, "Inicio pasada 3"=w1123) -> ("refnum out 2"=w1130:refnum<file>, "Refnum out"=w1131:refnum<k20>, "Buffer Underflow 2"=w1122:bool, "error out 4"=w1116:errorcluster, "Buffer Overflow 2"=w1121:bool, "error out"=w1115:errorcluster)  [unwired: 3 in]
                      n562 = local write "Buffer Overflow"(w1121) -> ()
                      n563 = call "Reporting_error.vi"("error out 2"=w1116, "Concept"="FPGA ") -> ("Reporting"=w1118:string)  [unwired: 1 in]
                      n564 = local read "Report"() -> (w1119:string)
                      n565 = local write "Buffer Underflow"(w1122) -> ()
                      n566 = Concatenate Strings(w1118, w1119) -> (w1117:string)
                      n567 = local write "Report"(w1117) -> ()
                    }
                    frame #3 {
                      n568 = xnode "Read/Write Control"("FPGA VI Reference In"=w1141, "error in"=w1140, "Stop"=TRUE ("stop")) -> ("FPGA VI Reference Out"=w1139:refnum<k20>, "error out"=w1138:errorcluster)
                      n569 = call "Reporting_error.vi"("error out 2"=w1132, "Concept"="Saving file ") -> ("Reporting"=w1135:string)  [unwired: 1 in]
                      n570 = Close File(refnum=w1142, error in=w1132) -> ()  [unwired: 2 out]
                      n571 = local read "Report"() -> (w1134:string)
                      n572 = xnode "Invoke Method"("FPGA VI Reference In"=w1139, "error in"=w1138) -> ("FPGA VI Reference Out"=w1144:refnum<k20>, "error out"=w1143:errorcluster)
                      n573 = Concatenate Strings(w1135, w1134) -> (w1136:string)
                      n574 = local write "Report"(w1136) -> ()
                    }
                  }
                }
              }
              frame #2 {
                n575 = local read "Frecuencia de muestreo (Hz)"() -> (w1168:dbl)
                n576 = local read "Nº de acelerómetros"() -> (w1159:i32)
                n577 = local read "Nº inductivos"() -> (w1158:i32)
                n578 = local read "Pattern amplitude (g)"() -> (w1160:dbl)
                n579 = local read "Pattern frequency (Hz)"() -> (w1161:dbl)
                n580 = local read "Folder"() -> (w1171:path)
                n581 = Add(x=w1159, y=w1158) -> (x+y=w1157:i32)
                n582 = call <vilib>:"Recursive File List.vi"("Folder Path"=w1171) -> ("All Files in Dir"=w1170:path[])  [unwired: 6 in, 4 out]
                n583 = local read "Report"() -> (w1153:string)
                n584 = call "Acel_calib_detector.vi"("Frecuencia\nmuestreo"=w1168, "Pattern frequency (Hz)"=w1161, "Nº canales"=w1157, "All Files in Dir"=w1170) -> ("Continue calibrating?"=w1152:bool, "Reporting"=w1167:string, "Acceler.\ndetected"=w1156:i32, "Acel Cal measurements"=w1169:sgl[][])
                n585 = Concatenate Strings(w1167, w1153) -> (w1154:string)
                n586 = local write "Report"(w1154) -> ()
                n587 = case shown="True" w1152 {
                  tunnel: w1169 -> [_ w1187]
                  tunnel: w1168 -> [_ w1185]
                  tunnel: [w1174 w1184] -> w1164
                  tunnel: [w1174 w1183] -> w1163
                  tunnel: [w1174 w1182] -> w1162
                  tunnel: w1161 -> [_ w1181]
                  tunnel: w1160 -> [_ w1180]
                  tunnel: [-1.0 ("Calibration parameter") w1179] -> w1155
                  frame False {
                    w1174 = "" ("Reporting2")
                  }
                  frame True {
                    n588 = local read "Report"() -> (w1177:string)
                    n589 = call "Acel_calib_frequency.vi"("Pattern frequency (Hz)"=w1181, "Frecuencia\nmuestreo"=w1185, "Acel Cal measurements in"=w1187) -> ("Valid frequency"=w1176:bool, "Reporting2"=w1184:string, "Acel Cal measurements out"=w1186:sgl[][])  [unwired: 1 in, 1 out]
                    n590 = Concatenate Strings(w1184, w1177) -> (w1178:string)
                    n591 = local write "Report"(w1178) -> ()
                    n592 = case shown="True" w1176 {
                      tunnel: w1186 -> [_ w1200]
                      tunnel: w1185 -> [_ w1199]
                      tunnel: [w1188 w1197] -> w1183
                      tunnel: [w1188 w1196] -> w1182
                      tunnel: w1181 -> [_ w1195]
                      tunnel: w1180 -> [_ w1194]
                      tunnel: [-1.0 ("Calibration parameter") w1193] -> w1179
                      frame False {
                        w1188 = "" ("Reporting 3")
                      }
                      frame True {
                        n593 = call "Acel_calib_noise_files_out.vi"("Pattern frequency (Hz)"=w1195, "Frecuencia\nmuestreo"=w1199, "Acel Cal measurements in"=w1200) -> ("Measurements OK"=w1190:bool, "Reporting 3"=w1197:string, "Acel Cal measurements out 2"=w1198:sgl[][])  [unwired: 6 in]
                        n594 = local read "Report"() -> (w1192:string)
                        n595 = Concatenate Strings(w1197, w1192) -> (w1191:string)
                        n596 = local write "Report"(w1191) -> ()
                        n597 = case shown="True" w1190 {
                          tunnel: w1199 -> [_ w1210]
                          tunnel: w1198 -> [_ w1209]
                          tunnel: ["" ("Reporting 4") w1208] -> w1196
                          tunnel: w1195 -> [_ w1207]
                          tunnel: w1194 -> [_ w1206]
                          tunnel: [-1.0 ("Calibration parameter") w1205] -> w1193
                          frame False {
                          }
                          frame True {
                            n598 = call "Acel_calib_calib.vi"("Acel Cal measurements in"=w1209, "Frecuencia\nmuestreo"=w1210, "Pattern frequency (Hz)"=w1207, "Pattern\namplitude"=w1206) -> ("Calibration parameter"=w1205:dbl, "Reporting 4"=w1208:string)  [unwired: 7 in, 3 out]
                            n599 = local read "Report"() -> (w1203:string)
                            n600 = Concatenate Strings(w1208, w1203) -> (w1204:string)
                            n601 = local write "Report"(w1204) -> ()
                          }
                        }
                      }
                    }
                  }
                }
                n602 = local read "calibration log"() -> (w1165:path)
                n603 = Concatenate Strings(w1167, w1164, w1163, w1162) -> (w1166:string)
                n604 = Write to Text File(file (use dialog)=w1165, text=w1166) -> ()  [unwired: 2 in, 3 out]
              }
              frame #3 {
                n605 = local read "Save calibration"() -> (w1212:bool)
                n606 = Add(x=w1215, y=8) -> (x+y=w1213:i32)
                n607 = case shown="True" w1212 {
                  tunnel: w1213 -> [_ w1227]
                  tunnel: w1211 -> [_ w1220]
                  frame False {
                  }
                  frame True {
                    w1228 = "Parametros"  # Key 1
                    n608 = local read "configuration file path"() -> (w1221:path)
                    n609 = Number To Decimal String(number=w1227) -> (decimal integer string=w1229:string)  [unwired: 1 in]
                    n610 = Concatenate Strings(w1228, w1229) -> (w1219:string)
                    n611 = call <vilib>:"Open Config Data.vi"("create file if necessary (T)"=TRUE, "configuration file path"=w1221) -> ("error out"=w1222:errorcluster, "refnum"=w1223:T11)  [unwired: 1 in, 7 out]
                    n612 = call-poly <vilib>:"Write Key.vi"("section"="Adquisicion", "error in (no error)"=w1222, "value"=w1220, "key"=w1219, "refnum"=w1223) -> ("error out"=w1226:errorcluster, "refnum out"=w1225:T11)  [unwired: 3 in, 2 out]
                    n613 = call <vilib>:"Close Config Data.vi"("error in (no error)"=w1226, "refnum"=w1225) -> ()  [unwired: 8 in, 2 out]
                  }
                }
              }
            }
          }
        }
        "error manipulacion archivos" <- w96
        n614 = local read "Parar la aplicación"() -> (w94:bool)
      }
      n615 = xnode "Close FPGA VI Reference"("FPGA VI Reference In"=w86, "error in"=w85) -> ("error out"=→"error FPGA":errorcluster)
    }
    frame #3 {
      n616 = local read "RFID_ID"() -> (w1238:refnum<k5>)
      n617 = call "LH6HD.vi"("Action"=enum16{"Init", "Start", "Read", "Stop", "Exit"}."Stop") -> ("error out"=→"RFID_LR6_Error":errorcluster)  [unwired: 9 in, 1 out]
      n618 = TCP Close Connection(connection ID=w1238) -> (error out=→"RFID_Error":errorcluster)  [unwired: 1 in, 2 out]
    }
  }
